vi "2017RefLoopPulseGen_Summer.vi"() -> ()   [LabVIEW 2015]
uses:
  Utility Sub VIs/pulse_generator_controls_multiheater_refnums.ctl
  Stop_Global_Variable.vi
  Utility Sub VIs/pulse_generator_data_controls_refnums.ctl
  Utility Sub VIs/pulse_generator_data_refnums.ctl
  Utility Sub VIs/pulse_generator_data_charts_refnums.ctl
  <vilib>/addons/control/pid/NI_PID_autopid.lvlib
  <vilib>/Utility/error.llb/DialogType.ctl
  <vilib>/DAQmx/configure/task.llb/DAQmx Configure Watchdog Expiration States (Counter Output).vi
  <vilib>/DAQmx/read.llb/DAQmx Read (Analog 1D Wfm NChan NSamp).vi
  <vilib>/DAQmx/configure/task.llb/DAQmx Configure Watchdog Expiration States (Analog Output).vi
  Utility Sub VIs/pulse_generator_data.ctl
  Utility Sub VIs/pulse_generator_data_controls.ctl
  Utility Sub VIs/pulse_generator_data_charts.ctl
  Utility Sub VIs/pulse_generator_multiheater_controls.ctl
  Input Channel Lists/test_section_physical_channels.ctl
  Input Channel Lists/pg_control_physical_channels.ctl
  Input Channel Lists/watchdog_config_channels.ctl
  Input Channel Lists/valve_physical_channels.ctl
  Utility Sub VIs/valve_pid_control.ctl
  Input Channel Lists/float_switch_physical_channels.ctl
  Input Channel Lists/pulse_generator_input_physical_channels.ctl
panel:
  out "dP Queue":refnum<queue>
  out "loopDataQueue":refnum<queue>
  out "Float 4":bool
  out "Float 3":bool
  out "Float 2":bool
  out "Float 1":bool
  out "Pulse Generator":u8(slide) scale=0.0..100.0 scale format="%.0f%"
  out "autoOffsetPsatQueue":refnum<queue>
  out "start time":timestamp
  out "Seconds Since\nSession Start":dbl
  out "dP Recording Progress":u32(slide) scale=0.0..10000.0
  out "dP Data Index":dbl
  out "Loop Data Index":dbl
  in  "dP Data Prefix":string
  in  "dP Data Folder":path
  in  "Loop Data Prefix":string
  in  "Loop Data Folder":path
  in  "Record dP Data":bool
  in  "Record Loop Data":bool
  out "dP Data Labels":string[](array[string])=["Vap Mass Flow", "Liq Mass Flow", "DP", "Liq Tank P", "LiqTank T", "Sep P", "SepT", "Liq In P", "Liq In T", "Vap Tank P", "Vap Tank T", "Dev Section P", "Dev Section T", "Up TS P", "Up TS T", "Low TS P", "Low TS T", "Cond Top T", "Evap Top T", "Cond Bot T", "Evap Bot T", "Win 3-4 P", "Top Heat T", "Bot Heat T"]
  out "Time Stamp":timestamp format="%<%H:%M:%S%1u>T"
  out "Loop Data Labels":string[](array[string])=["Vap Mass Flow", "Liq Mass Flow", "DP", "Liq Tank P", "LiqTank T", "Sep P", "SepT", "Liq In P", "Liq In T", "Vap Tank P", "Vap Tank T", "Dev Section P", "Dev Section T", "Up TS P", "Up TS T", "Low TS P", "Low TS T", "Cond Top T", "Evap Top T", "Cond Bot T", "Evap Bot T", "Win 3-4 P", "Top Heat T", "Bot Heat T"]
  in  "Tab Control":T1(tab)
  out "Auto Offset Progress":u32(slide) scale=0.0..20.0
  out "Pressure/Temperature/Mixture Properties":T2
  in  "Offset Parameters":T3={"Separator \nTemperature"=0.0, "Separator Pressure"=0.0, "Lower Test Section\nTemperature"=0.0, "Lower Test Section\nPressure"=0.0, "Vapor Tank (Top) \nHeater"=0.0, "Liquid Tank (Bottom) \nHeater"=0.0, "Vapor Tank\nTemperature Offset"=0.0, "Vapor Tank\nPressure "=0.0, "Upper Test Section\nTemperature"=0.0, "Upper Test Section\nPressure"=0.0, "Vapor Inlet \nTemperature"=0.0, "Dev Section\nPressure"=0.0, "Liquid Tank\nTemperature"=0.0, "Liquid Tank\nPressure"=0.0, "Liquid Inlet\nTemperature "=0.0, "Liquid Inlet\nPressure"=0.0, "Atmospheric Pressure [Pa]"=101325.0}
  in  "Auto Offset":bool
  out "# of Averages Processed":i32
  out "Dynamic Data Type":dynamicdata(graph)
  out "Vapor Mass Flow Rate":dynamicdata(graph)
  out "Liquid Mass Flow Rate":dynamicdata(graph)
  out "Vapor Flow Data":T4
  out "Liquid Flow Data":T5
  in  "Liquid PID Control":T6={"proportional gain (Kc)"=1.0, "integral time (Ti, min)"=0.01, "derivative time (Td, min)"=0.0, "Valve Voltage [V]"=0.0, "Min % Open"=2.0, "Max % Open"=3.0, "Reinitialize?"=FALSE, "Valve On/Off"=FALSE, "Mode"=FALSE, "Full Flow Rate"=0.0, "Flow Set Point [g/s]"=0.0, "AutoTune"=FALSE} {"Flow Set Point [g/s]" format="%.2f"; "Full Flow Rate" format="%.2f"; "Max % Open" min=0.0 max=100.0 format="%.2f"; "Min % Open" min=0.0 max=100.0 format="%.2f"; "Valve Voltage [V]" format="%.2f"; "derivative time (Td, min)" format="%.3f"; "integral time (Ti, min)" format="%.3f"; "proportional gain (Kc)" format="%.3f"}
  in  "Vapor PID Control":T6={"proportional gain (Kc)"=1.0, "integral time (Ti, min)"=0.01, "derivative time (Td, min)"=0.0, "Valve Voltage [V]"=0.0, "Min % Open"=2.0, "Max % Open"=3.0, "Reinitialize?"=FALSE, "Valve On/Off"=FALSE, "Mode"=FALSE, "Full Flow Rate"=0.0, "Flow Set Point [g/s]"=0.0, "AutoTune"=FALSE} {"Flow Set Point [g/s]" format="%.2f"; "Full Flow Rate" format="%.2f"; "Max % Open" min=0.0 max=100.0 format="%.2f"; "Min % Open" min=0.0 max=100.0 format="%.2f"; "Valve Voltage [V]" format="%.2f"; "derivative time (Td, min)" format="%.3f"; "integral time (Ti, min)" format="%.3f"; "proportional gain (Kc)" format="%.3f"}
  in  "Pulse Generator Offsets & Data Saving Controls":T7={"PG-TS Offset"=11500.0, "Pitot Offset"=0.0, "PG Abs Offset"=11500.0, "Sampling\nFrequency"=1000.0, "Recording Duration"=10.0}
  out "Pulse Generator Measurements":T8={"PG to TS dP"=4351.8068090218785, "PG Abs"=119484.80284900061, "Mass Flow Rate"=nan, "Pitot dP"=-4308.9404273994505, "Pitot Amps"=2.6415199999999147e-07, "Vapor Temperature"=19.805676371442082, "Liquid Temperature"=19.52526901660894, "Vapor Sat Pressure"=121.24568157832624, "Liquid Sat Pressure"=119.96937909943745, "W1-4 dP[Pa]"=19.52526901660894, "W1-7 dP[Pa]"=119.96937909943745}
  out "Pulse Generator Charts":T9={" Camera Voltage"=9.650720988784618, "Pitot dP"=-0.0006103608758678569, "Absolute Tank Pressure"=119484.80284900061, "Pulse Generator to Test Section dP"=11360.460004869077}
  in  "Commit Settings":bool
  in  "Settings Subpanel":enum32{"Input", "Output", "Safety"}(tab)
  in  "Input":T13={"Test Section Physical Channels"={"Vapor Mass Flow Current"="cDAQ1Mod1/ai10", "Vapor Line Density Current"="cDAQ1Mod1/ai11", "Liquid Mass Flow Current"="cDAQ1Mod1/ai8", "Liquid Line Density Current"="cDAQ1Mod1/ai9", "Vapor Tank Pressure"="cDAQ1Mod1/ai3", "Liquid Tank Pressure"="cDAQ1Mod1/ai2", "Separator Pressure"="cDAQ1Mod1/ai4", "Liquid Inlet Pressure"="cDAQ1Mod1/ai0", "Dev Section Pressure"="cDAQ1Mod1/ai1", "Vapor Tank Temperature"="cDAQ1Mod6/ai2", "Vapor Inlet Temperature"="cDAQ1Mod6/ai0", "Liquid Tank Temperature"="cDAQ1Mod6/ai3", "Liquid Inlet Temperature"="cDAQ1Mod6/ai4", "Separator Temperature"="cDAQ1Mod6/ai1", "Lower Test Section Pressure"="cDAQ1Mod1/ai5", "Lower Test Section Temperature"="cDAQ1Mod6/ai5", "Top Heater Temperature"="cDAQ1Mod6/ai6", "Bottom Heater Temperature"="cDAQ1Mod6/ai7", "Pressure Drop"="cDAQ1Mod1/ai12", "Upper Test Section Temperature"="cDAQ1Mod6/ai9", "Upper Test Section Pressure"="cDAQ1Mod1/ai7", "Condenser Top Temperature"="cDAQ1Mod6/ai8", "Condenser Bottom Temperature"="cDAQ1Mod6/ai10", "Evaporator Top Temperature"="cDAQ1Mod6/ai11", "Evaporator Bottom Temperature"="cDAQ1Mod6/ai12", "Test Section Window 3-4 Pressure"="cDAQ1Mod1/ai6"}, "Float Switch Physical Channels"={"Float Line 1"="", "Float Line 2"="", "Float Line 3"="", "Float Line 4"=""}, "Pulse Generator Input Physical Channels"={"Absolute Pressure"="cDAQ1Mod5/ai1", "PG to TS dP"="cDAQ1Mod5/ai0", "Pitot dP"="cDAQ1Mod3/ai6", "PG Temperature 1"="cDAQ1Mod7/ai0", "PG Temperature 2"="cDAQ1Mod7/ai1", "dP Windows 1 to 7"="cDAQ1Mod1/ai2", "dP Windows 1 to 4"="cDAQ1Mod3/ai3", "Camera Votlage"="cDAQ1Mod2/ai0"}}
  in  "Output":T16={"Pulse Generator Control Physical Channels"={"1000W 1"="Dev1/port1/line0", "1000W 2"="Dev1/port1/line1", "1000W 3"="Dev1/port1/line2", "500W 1"="Dev1/port1/line3", "250W 1"="cDAQ1Mod8/ctr0", "125W 1 Var"="cDAQ1Mod8/ctr0", "125W Variable/Fixed"="Fixed", "125W 1 Fix"="cDAQ1Mod8/ctr0", "Counter Line"="cDAQ1Mod8/ctr0", "Direction Line"="cDAQ1Mod8/ctr0"}, "Vapor/Liquid Valve Physical Channels"={"Vapor Valve"="cDAQ1Mod4/ao2", "Liquid Valve"="cDAQ1Mod4/ao3"}}
  in  "Safety":T17
  in  "Watchdog Configurations":T18 {"Counter Outputs"."expiration state" items=["Low"=10214, "High"=10192, "No Change"=10160]; "Analog Outputs"."output type" items=["Voltage"=10322, "Current"=10134, "No Change"=10160]; "Digital Outputs"."expiration state" items=["High"=10192, "Low"=10214, "Tristate"=10310, "No Change"=10160]}
  out "System Running":bool
  in  "Pulse Train, Steam Heater Controls":T19={"Start Pulse"=FALSE, "Stop Pulse"=FALSE, "Pulse Gen\nActive?"=FALSE, "Frequency (Hz)"=3000.0, "Duty Cycle"=0.5, "Idle State"=10214, "Steps"=1000, "Stepper Motor Direction"=FALSE, "Heaters"=FALSE, "Heater ON?"=FALSE, "1000-1"=FALSE, "1000-2"=FALSE, "1000-3"=FALSE, "500-1"=FALSE, "250-1"=FALSE, "125W Duty Cycle"=0.5, "125W Frequency (Hz)"=1000.0, "125-1"=FALSE} {"125W Frequency (Hz)" min=0.0; "125W Duty Cycle" min=0.0; "Frequency (Hz)" min=1.0 step=500.0; "Duty Cycle" min=0.1 max=0.99 step=0.1; "Idle State" items=["High"=10192, "Low"=10214]}
  out "error out":errorcluster
  out "Loop Time [ms]":u32
  in  "Stop":bool
  # "Saturation\nPressure [Pa]"
  # "Saturation\nTemperature [C]"
  # "Pressure [Pa]"
  # "Temperature [C]"
  # "Streamwise(dP)"
  # "Liquid Tank"
  # "Separator"
  # "Liquid Inlet"
  # "Vapor Tank"
  # "Vapor Inlet\n(Dev Section)"
  # "Upper Test Section"
  # "Lower Test Section"
  # "Offsets"
  # "Pulse Generator - Test Section dP"
  # "Pulse Generator Absolute Pressure"
  # "Pitot dP"
  # "Pitot Current"
  # "Mass Flow Rate"
  # "Heater Lines and Switches"
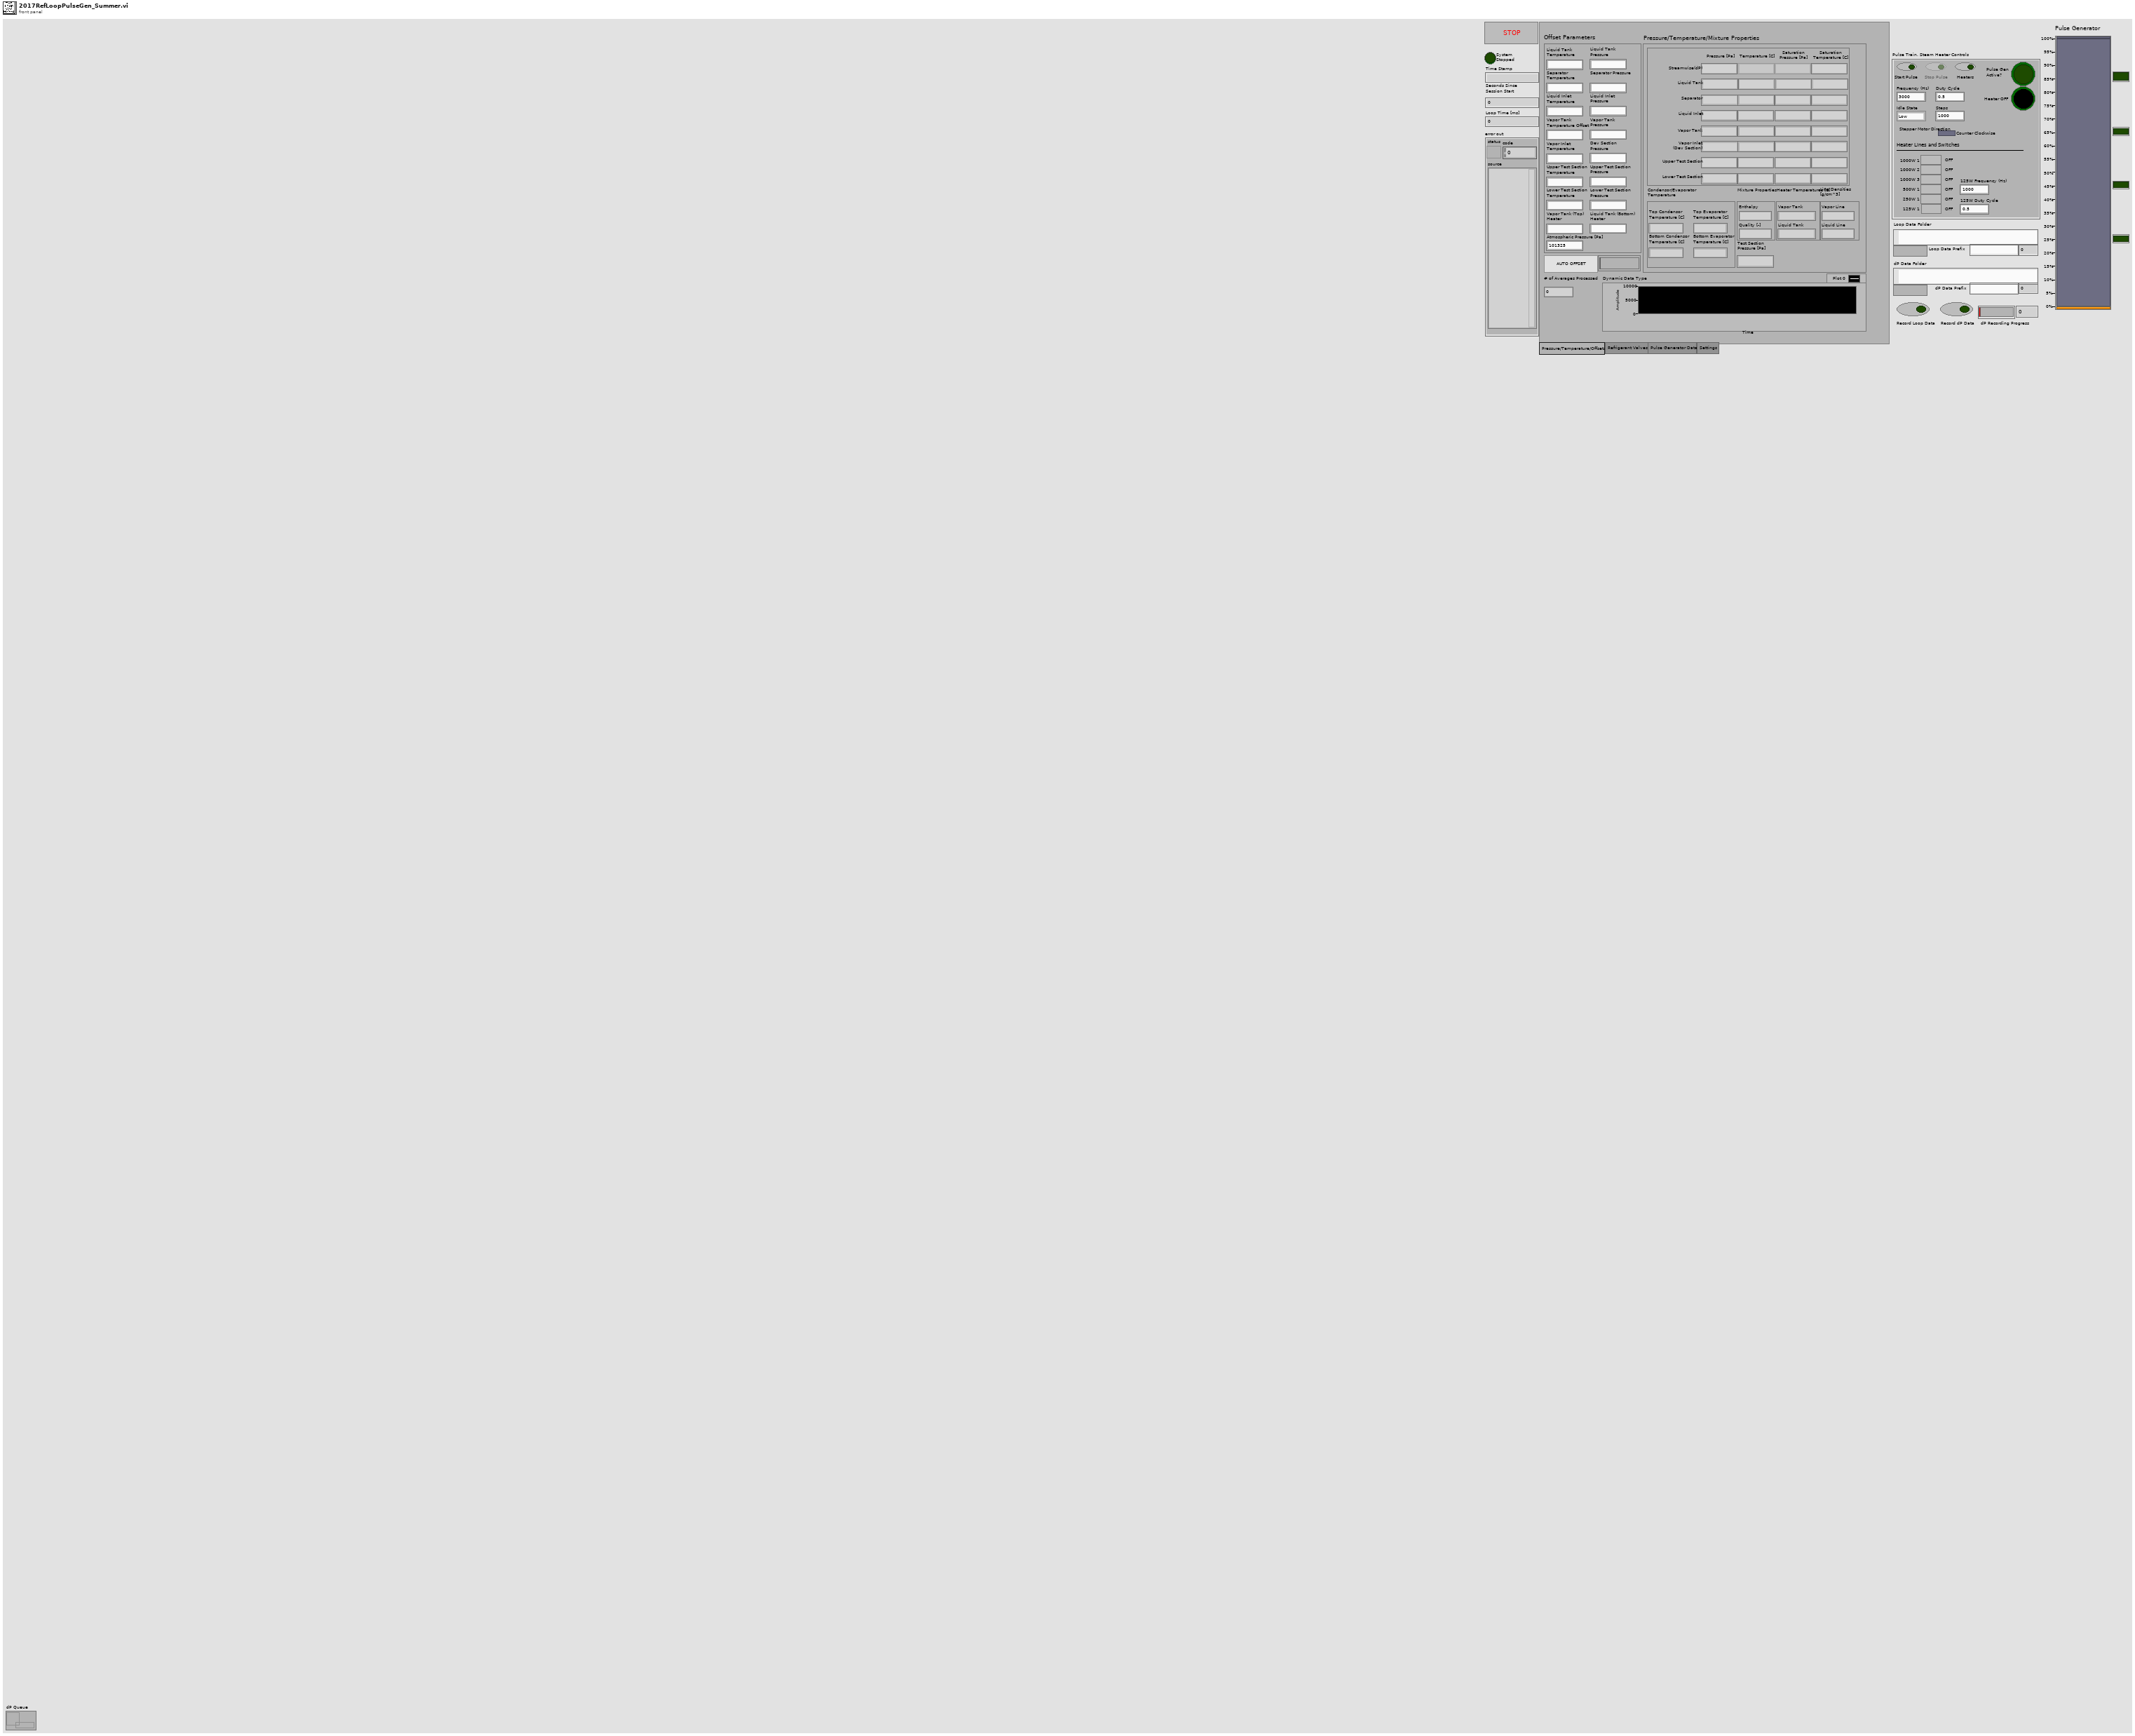
[diagram p1: front panel]
types:
  T1 = enum32{"Pressure/Temperature/Offsets", "Refrigerant Valves", "Pulse Generator Data", "Settings"}
  T2 = cluster{"Line Densities\n[g/cm^3]":cluster{"Vapor Line":dbl, "Liquid Line":dbl}, "Mixture Properties":cluster{"Enthalpy":dbl, "Quality [-]":dbl}, "[Readings]":cluster{"Streamwise P":dbl, "Streamwise T":dbl, "Streamwise Sat P":dbl, "Streamwise Sat T":dbl, "Liquid Tank P":dbl, "Liquid Tank T":dbl, "Liquid Tank Sat P":dbl, "Liquid Tank Sat T":dbl, "Separator P":dbl, "Separator T":dbl, "Separator Sat P":dbl, "Separator Sat T":dbl, "Liquid Inlet P":dbl, "Liquid Inlet T":dbl, "Liquid Inlet Sat P":dbl, "Liquid Inlet Sat T":dbl, "Vapor Tank P":dbl, "Vapor Tank T":dbl, "Vapor Tank Sat P":dbl, "Vapor Tank Sat T":dbl, "Vapor Inlet P":dbl, "Vapor Inlet T":dbl, "Vapor Inlet Sat P":dbl, "Vapor Inlet Sat T":dbl, "Upper Test Section P":dbl, "Upper Test Section T":dbl, "Upper Test Section Sat P":dbl, "Upper Test Section Sat T":dbl, "Lower Test Section P":dbl, "Lower Test Section T":dbl, "Lower Test Section Sat P":dbl, "Lower Test Section Sat T":dbl}, "Condensor/Evaporator\nTemperature":cluster{"Bottom Evaporator\nTemperature [C]":dbl, "Bottom Condensor\nTemperature [C]":dbl, "Top Evaporator\nTemperature [C]":dbl, "Top Condensor\nTemperature [C]":dbl}, "Test Section \nPressure [Pa]":dbl, "Heater Temperatures [C]":cluster{"Vapor Tank":dbl, "Liquid Tank":dbl}}
  T3 = cluster{"Separator \nTemperature":dbl, "Separator Pressure":dbl, "Lower Test Section\nTemperature":dbl, "Lower Test Section\nPressure":dbl, "Vapor Tank (Top) \nHeater":dbl, "Liquid Tank (Bottom) \nHeater":dbl, "Vapor Tank\nTemperature Offset":dbl, "Vapor Tank\nPressure ":dbl, "Upper Test Section\nTemperature":dbl, "Upper Test Section\nPressure":dbl, "Vapor Inlet \nTemperature":dbl, "Dev Section\nPressure":dbl, "Liquid Tank\nTemperature":dbl, "Liquid Tank\nPressure":dbl, "Liquid Inlet\nTemperature ":dbl, "Liquid Inlet\nPressure":dbl, "Atmospheric Pressure [Pa]":dbl}
  T4 = cluster{"Vapor Flow rate [g/s]":dbl, "Line Density [g/cm^3]":dbl}
  T5 = cluster{"Liquid Flow rate [g/s]":dbl, "Line Density [g/cm^3]":dbl}
  T6 = typedef "valve_pid_control.ctl" = cluster{"proportional gain (Kc)":dbl, "integral time (Ti, min)":dbl, "derivative time (Td, min)":dbl, "Valve Voltage [V]":dbl, "Min % Open":dbl, "Max % Open":dbl, "Reinitialize?":bool, "Valve On/Off":bool, "Mode":bool, "Full Flow Rate":dbl, "Flow Set Point [g/s]":dbl, "AutoTune":bool}
  T7 = typedef "pulse_generator_data_controls.ctl" = cluster{"PG-TS Offset":dbl, "Pitot Offset":dbl, "PG Abs Offset":dbl, "Sampling\nFrequency":dbl, "Recording Duration":dbl}
  T8 = typedef "pulse_generator_data.ctl" = cluster{"PG to TS dP":dbl, "PG Abs":dbl, "Mass Flow Rate":dbl, "Pitot dP":dbl, "Pitot Amps":dbl, "Vapor Temperature":dbl, "Liquid Temperature":dbl, "Vapor Sat Pressure":dbl, "Liquid Sat Pressure":dbl, "W1-4 dP[Pa]":dbl, "W1-7 dP[Pa]":dbl}
  T9 = typedef "pulse_generator_data_charts.ctl" = cluster{" Camera Voltage":dbl, "Pitot dP":dbl, "Absolute Tank Pressure":dbl, "Pulse Generator to Test Section dP":dbl}
  T10 = typedef "test_section_physical_channels.ctl" = cluster{"Vapor Mass Flow Current":tag, "Vapor Line Density Current":tag, "Liquid Mass Flow Current":tag, "Liquid Line Density Current":tag, "Vapor Tank Pressure":tag, "Liquid Tank Pressure":tag, "Separator Pressure":tag, "Liquid Inlet Pressure":tag, "Dev Section Pressure":tag, "Vapor Tank Temperature":tag, "Vapor Inlet Temperature":tag, "Liquid Tank Temperature":tag, "Liquid Inlet Temperature":tag, "Separator Temperature":tag, "Lower Test Section Pressure":tag, "Lower Test Section Temperature":tag, "Top Heater Temperature":tag, "Bottom Heater Temperature":tag, "Pressure Drop":tag, "Upper Test Section Temperature":tag, "Upper Test Section Pressure":tag, "Condenser Top Temperature":tag, "Condenser Bottom Temperature":tag, "Evaporator Top Temperature":tag, "Evaporator Bottom Temperature":tag, "Test Section Window 3-4 Pressure":tag}
  T11 = typedef "float_switch_physical_channels.ctl" = cluster{"Float Line 1":tag, "Float Line 2":tag, "Float Line 3":tag, "Float Line 4":tag}
  T12 = typedef "pulse_generator_input_physical_channels.ctl" = cluster{"Absolute Pressure":tag, "PG to TS dP":tag, "Pitot dP":tag, "PG Temperature 1":tag, "PG Temperature 2":tag, "dP Windows 1 to 7":tag, "dP Windows 1 to 4":tag, "Camera Votlage":tag}
  T13 = cluster{"Test Section Physical Channels":T10, "Float Switch Physical Channels":T11, "Pulse Generator Input Physical Channels":T12}
  T14 = typedef "pg_control_physical_channels.ctl" = cluster{"1000W 1":tag, "1000W 2":tag, "1000W 3":tag, "500W 1":tag, "250W 1":tag, "125W 1 Var":tag, "125W Variable/Fixed":string, "125W 1 Fix":tag, "Counter Line":tag, "Direction Line":tag}
  T15 = typedef "valve_physical_channels.ctl" = cluster{"Vapor Valve":tag, "Liquid Valve":tag}
  T16 = cluster{"Pulse Generator Control Physical Channels":T14, "Vapor/Liquid Valve Physical Channels":T15}
  T17 = cluster{"Pulse Generator Safety Values":cluster{"Absolute Pulse Generator Pressure Limit":dbl, "Seconds Allowed Pulse Generator Excess Pressure":dbl, "Absolute Pulse Generator Temperature Limit":dbl}}
  T18 = typedef "watchdog_config_channels.ctl" = cluster{"Task Name":string, "DAQmx Device Name":tag, "Digital Outputs":cluster{"physical channel":tag, "expiration state":u16}[], "Analog Outputs":cluster{"physical channel":tag, "value":dbl, "output type":i32}[], "Counter Outputs":cluster{"physical channel":tag, "expiration state":u16}[]}[]
  T19 = typedef "pulse_generator_multiheater_controls.ctl" = cluster{"Start Pulse":bool, "Stop Pulse":bool, "Pulse Gen\nActive?":bool, "Frequency (Hz)":dbl, "Duty Cycle":dbl, "Idle State":i32, "Steps":i32, "Stepper Motor Direction":bool, "Heaters":bool, "Heater ON?":bool, "1000-1":bool, "1000-2":bool, "1000-3":bool, "500-1":bool, "250-1":bool, "125W Duty Cycle":dbl, "125W Frequency (Hz)":dbl, "125-1":bool}
  T20 = cluster{"Vapor Flow rate [g/s]":dbl, "Liquid Flow rate [g/s]":dbl, "Pressure/Temperature/Mixture Properties":cluster{"Line Densities\n[g/cm^3]":cluster{"Vapor Line":dbl, "Liquid Line":dbl}, "Mixture Properties":cluster{"Enthalpy":dbl, "Quality [-]":dbl}, "[Readings]":cluster{"Streamwise P":dbl, "Streamwise T":dbl, "Streamwise Sat P":dbl, "Streamwise Sat T":dbl, "Liquid Tank P":dbl, "Liquid Tank T":dbl, "Liquid Tank Sat P":dbl, "Liquid Tank Sat T":dbl, "Separator P":dbl, "Separator T":dbl, "Separator Sat P":dbl, "Separator Sat T":dbl, "Liquid Inlet P":dbl, "Liquid Inlet T":dbl, "Liquid Inlet Sat P":dbl, "Liquid Inlet Sat T":dbl, "Vapor Tank P":dbl, "Vapor Tank T":dbl, "Vapor Tank Sat P":dbl, "Vapor Tank Sat T":dbl, "Vapor Inlet P":dbl, "Vapor Inlet T":dbl, "Vapor Inlet Sat P":dbl, "Vapor Inlet Sat T":dbl, "Upper Test Section P":dbl, "Upper Test Section T":dbl, "Upper Test Section Sat P":dbl, "Upper Test Section Sat T":dbl, "Lower Test Section P":dbl, "Lower Test Section T":dbl, "Lower Test Section Sat P":dbl, "Lower Test Section Sat T":dbl}, "Condensor/Evaporator\nTemperature":cluster{"Bottom Evaporator\nTemperature [C]":dbl, "Bottom Condensor\nTemperature [C]":dbl, "Top Evaporator\nTemperature [C]":dbl, "Top Condensor\nTemperature [C]":dbl}, "Test Section \nPressure [Pa]":dbl, "Heater Temperatures [C]":cluster{"Vapor Tank":dbl, "Liquid Tank":dbl}}, "Seconds Since \nSession Start":dbl}
  T21 = enum8{"Enabled", "Disabled", "Disabled and Grayed Out"}
  T22 = typedef "DialogType.ctl" = u16
  T23 = cluster{"physical channel":tag, "expiration state":u16}[]
  T24 = cluster{"physical channel":tag, "value":dbl, "output type":i32}[]
  T25 = cluster{"Vapor Flow rate [g/s]":dbl, "Liquid Flow rate [g/s]":dbl, "Pressure/Temperature/Mixture Properties":cluster{"Line Densities\n[g/cm^3]":cluster{"Vapor Line":dbl, "Liquid Line":dbl}, "Mixture Properties":cluster{"Enthalpy":dbl, "Quality [-]":dbl}, "[Readings]":cluster{"Streamwise P":dbl, "Streamwise T":dbl, "Streamwise Sat P":dbl, "Streamwise Sat T":dbl, "Liquid Tank P":dbl, "Liquid Tank T":dbl, "Liquid Tank Sat P":dbl, "Liquid Tank Sat T":dbl, "Separator P":dbl, "Separator T":dbl, "Separator Sat P":dbl, "Separator Sat T":dbl, "Liquid Inlet P":dbl, "Liquid Inlet T":dbl, "Liquid Inlet Sat P":dbl, "Liquid Inlet Sat T":dbl, "Vapor Tank P":dbl, "Vapor Tank T":dbl, "Vapor Tank Sat P":dbl, "Vapor Tank Sat T":dbl, "Vapor Inlet P":dbl, "Vapor Inlet T":dbl, "Vapor Inlet Sat P":dbl, "Vapor Inlet Sat T":dbl, "Upper Test Section P":dbl, "Upper Test Section T":dbl, "Upper Test Section Sat P":dbl, "Upper Test Section Sat T":dbl, "Lower Test Section P":dbl, "Lower Test Section T":dbl, "Lower Test Section Sat P":dbl, "Lower Test Section Sat T":dbl}, "Condensor/Evaporator\nTemperature":cluster{"Bottom Evaporator\nTemperature [C]":dbl, "Bottom Condensor\nTemperature [C]":dbl, "Top Evaporator\nTemperature [C]":dbl, "Top Condensor\nTemperature [C]":dbl}, "Test Section \nPressure [Pa]":dbl, "Heater Temperatures [C]":cluster{"Vapor Tank":dbl, "Liquid Tank":dbl}}, "Seconds Since\nSession Start":dbl}
  T26 = cluster{"proportional gain (Kc)":dbl, "integral time (Ti, min)":dbl, "derivative time (Td, min)":dbl}
  T27 = typedef "pulse_generator_data_charts_refnums.ctl" = cluster{"Pulse Generator to Test Section dP":refnum<vi>, "Pitot dP":refnum<vi>, "Abs Tank Pressure":refnum<vi>, "Camera Voltage":refnum<vi>}
  T28 = typedef "pulse_generator_data_refnums.ctl" = cluster{"Vapor Temperature":refnum<vi>, "Vapor Sat Pressure":refnum<vi>, "Liquid Temperature":refnum<vi>, "Liquid Sat Pressure":refnum<vi>, "PG to TS dP":refnum<vi>, "Pitot Current":refnum<vi>, "Pitot dP":refnum<vi>, "Mass Flow Rate":refnum<vi>, "PG Abs Pressure":refnum<vi>, "W1-4 dP":refnum<vi>, "W1-7 dP":refnum<vi>}
  T29 = typedef "pulse_generator_data_controls_refnums.ctl" = cluster{"PG Abs Offset":refnum<vi>, "Pitot Offset":refnum<vi>, "PG-TS Offset":refnum<vi>, "Recording Duration":refnum<vi>, "Sampling Rate":refnum<vi>}
  T30 = typedef "pulse_generator_controls_multiheater_refnums.ctl" = cluster{"Start Pulse":refnum<vi>, "Stop Pulse":refnum<vi>, "Heaters":refnum<vi>, "Counter":refnum<vi>, "Frequency (Hz)":refnum<vi>, "Duty Cycle":refnum<vi>, "Idle State":refnum<vi>, "Pulse Generator Active":refnum<vi>, "Stepper Motor Direction":refnum<vi>, "Steps":refnum<vi>, "Direction Line":refnum<vi>, "1000-1 Line":refnum<vi>, "1000-2 Line":refnum<vi>, "1000-3 Line":refnum<vi>, "500-1 Line":refnum<vi>, "250-1 Line":refnum<vi>, "125-1 Line Var":refnum<vi>, "1000-1":refnum<vi>, "1000-2":refnum<vi>, "1000-3":refnum<vi>, "500-1":refnum<vi>, "250-1":refnum<vi>, "125-1":refnum<vi>, "125W Frequency (Hz)":refnum<vi>, "125W Duty Cycle":refnum<vi>, "Heater ON?":refnum<vi>, "125-1 Line Fix":refnum<vi>}
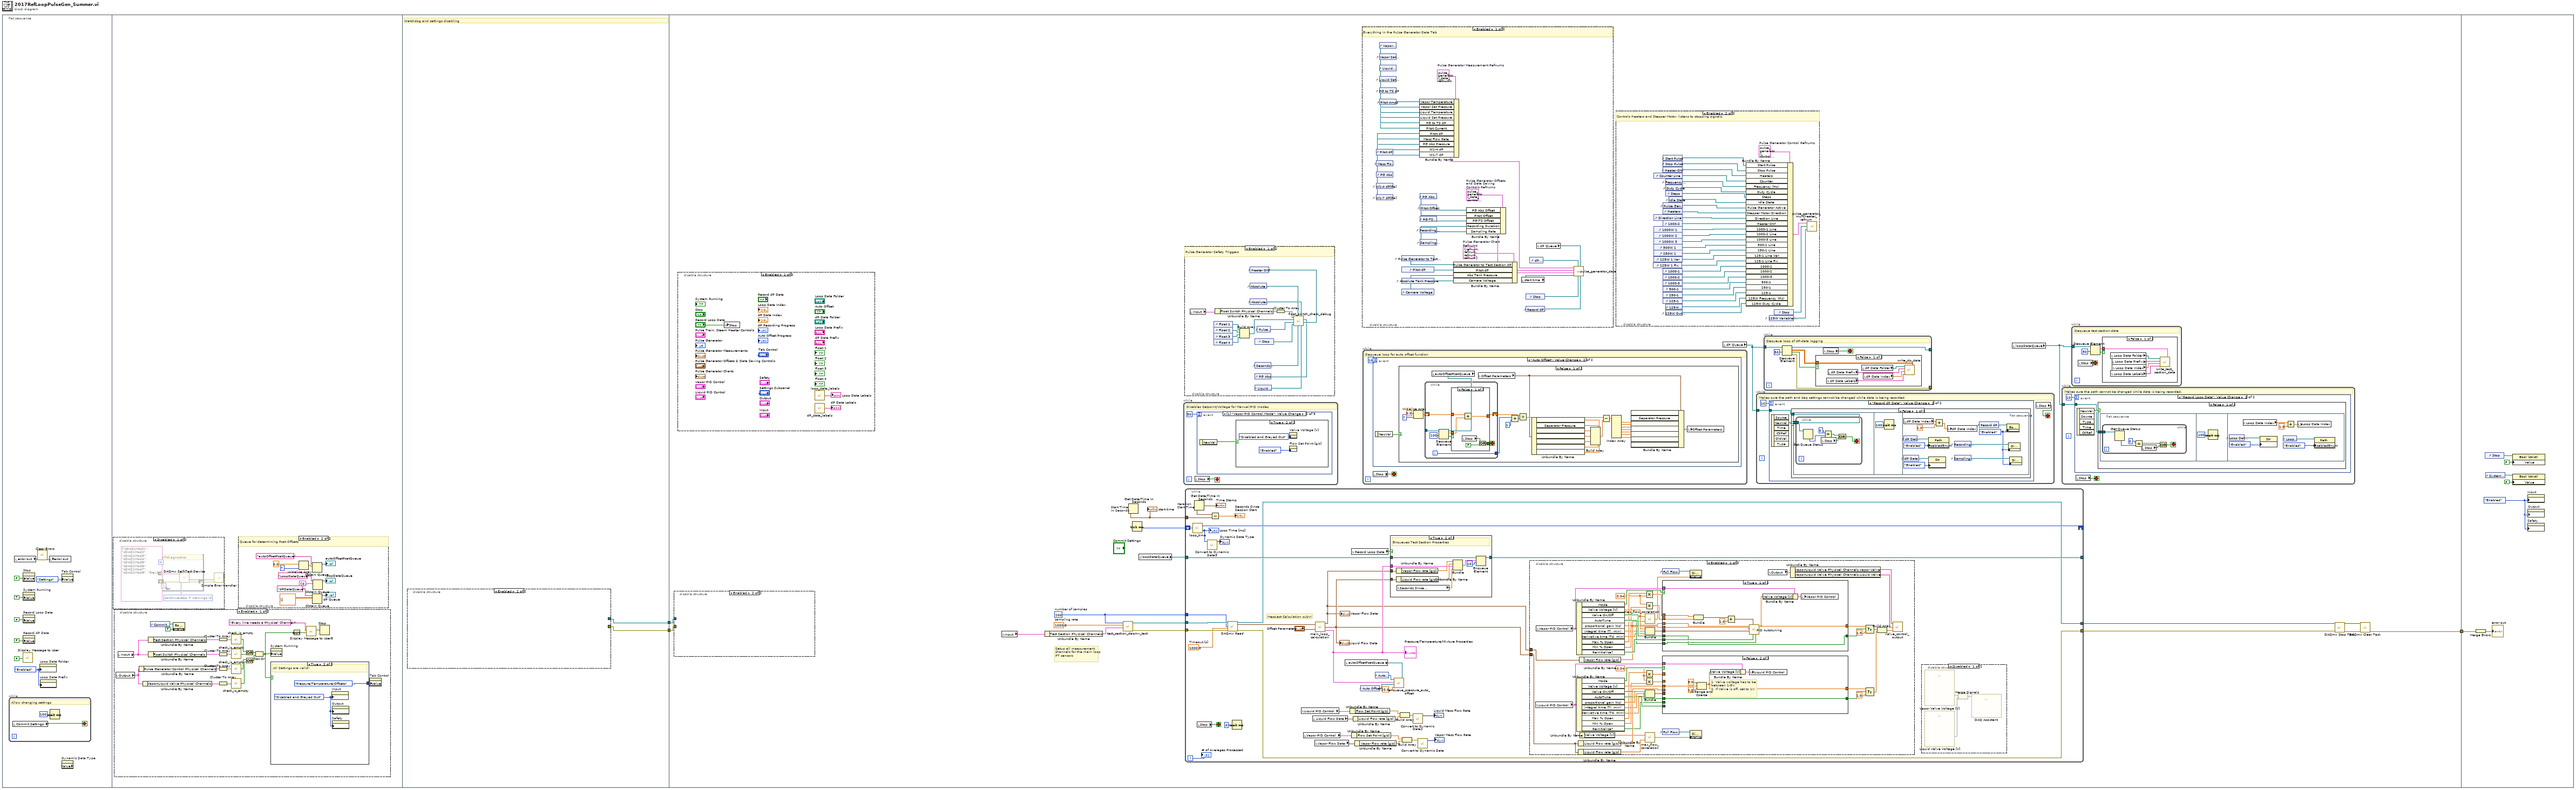
[diagram p0: block diagram]
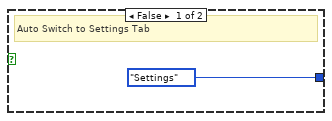
[diagram p3: hidden frame]
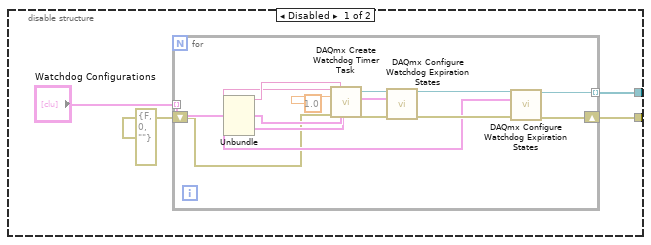
[diagram p6: hidden frame]
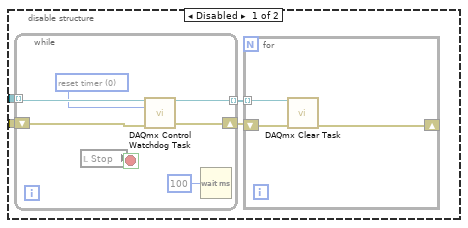
[diagram p11: hidden frame]
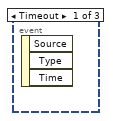
[diagram p12: hidden frame]
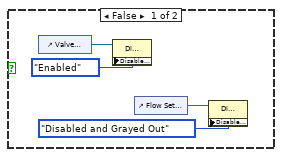
[diagram p13: hidden frame]
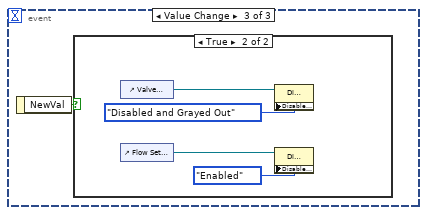
[diagram p14: hidden frame]
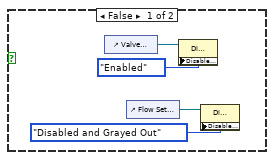
[diagram p15: hidden frame]
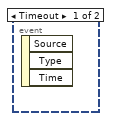
[diagram p16: hidden frame]
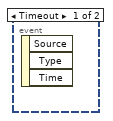
[diagram p19: hidden frame]
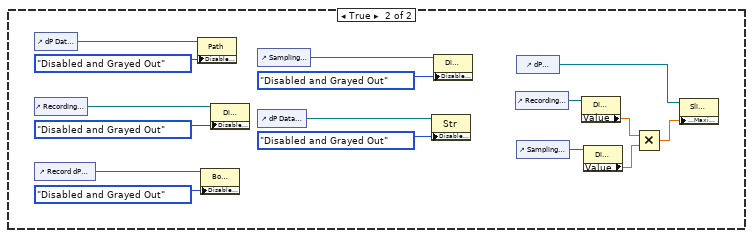
[diagram p20: hidden frame]
diagram:
  n1 = flat-sequence {
    tunnel: [w59] -> w2
    tunnel: [w58] -> w1
    tunnel: [w91] -> w3
    tunnel: w2 -> [w85]
    tunnel: w1 -> [w84]
    tunnel: w3 -> [w492]
    frame #0 {
      w4 = T21."Enabled" ("Disabled")
      n2 = while {
        stop <- w13 stop-if-true
        # "Allow changing settings"
        n3 = local read "Commit Settings"() -> (w13:bool)
        n4 = Wait (ms)(milliseconds to wait=u32 100) -> ()  [unwired: 1 out]
      }
      n5 = local read "error out"() -> (w12:errorcluster)
      n6 = call "Display Message to User"("Enable"=FALSE) -> ()  [unwired: 9 in, 2 out]
      n7 = property on="Stop" class="Bool (strict)"("Value"=FALSE) -> ()  [unwired: 2 in, 2 out]
      n8 = property on="System Running" class="Bool (strict)"("Value"=TRUE) -> ()  [unwired: 2 in, 2 out]
      n9 = property on="Record Loop Data" class="Bool (strict)"("Value"=FALSE) -> ()  [unwired: 2 in, 2 out]
      n10 = property on="Record dP Data" class="Bool (strict)"("Value"=FALSE) -> ()  [unwired: 2 in, 2 out]
      n11 = call <vilib>:"Clear Errors.vi"("error in (no error)"=w12) -> ("error out"=w10:errorcluster)  [unwired: 5 in, 1 out]
      n12 = property on="Loop Data Folder" class="Path"("DisabledEnum"=w4) -> ()  [unwired: 2 in, 2 out]
      n13 = property on="Loop Data Prefix" class="Str"("DisabledEnum"=w4) -> ()  [unwired: 2 in, 2 out]
      n14 = local write "error out"(w10) -> ()
      n15 = property on="Tab Control" class="TabCtl (strict)"("Value"=T1."Settings" ("Tab Control")) -> ()  [unwired: 2 in, 2 out]
      n16 = property on="Dynamic Data Type" class="WFChart (strict)" props=["Value"]() -> ()  [unwired: 2 in, 3 out]
    }
    frame #1 {
      n17 = disable-structure shown="Disabled" {
        frame Disabled {
          w52 = T22 4 items=["no dialog", "OK message", "continue or stop message", "OK message + warnings", "continue/stop + warnings"] ("type of dialog (OK msg:1)")
          n18 = for {
            tunnel: string[] ["cDAQ1Mod1", "cDAQ1Mod2", "cDAQ1Mod3", "cDAQ1Mod4", "cDAQ1Mod5", "cDAQ1Mod6", "cDAQ1Mod7", "cDAQ1Mod8", "Dev1"] -> [w57] mode=indexing
            shift-right: [w56] -> w53
            shift-left: _ -> [w55]
            # "Self-Diagnostics"
            n19 = call <vilib>:"DAQmx Self-Test Device.vi"("device in"=w57, "error in"=w55) -> ("error out"=w56:errorcluster)  [unwired: 13 in]
          }
          n20 = call <vilib>:"Simple Error Handler.vi"("type of dialog (OK msg:1)"=w52, "error in (no error)"=w53) -> ()  [unwired: 3 in, 5 out]
        }
        frame Enabled {
        }
      }
      n21 = disable-structure shown="Enabled" {
        frame Enabled {
          n22 = local read "Output"() -> (w26:T16)
          n23 = local read "Input"() -> (w32:T13)
          n24 = Unbundle By Name(w26) -> ("Pulse Generator Control Physical Channels"=w33:T14)
          n25 = Unbundle By Name(w26) -> ("Vapor/Liquid Valve Physical Channels"=w31:T15)
          n26 = Unbundle By Name(w32) -> ("Test Section Physical Channels"=w35:T10)
          n27 = Unbundle By Name(w32) -> ("Float Switch Physical Channels"=w34:T11)
          n28 = control-ref of="Commit Settings"() -> (w29:refnum<vi>)
          n29 = property class="Bool (strict)"(reference=w29, "Value"=FALSE ("Commit Settings")) -> ()  [unwired: 1 in, 2 out]
          n30 = Cluster To Array(cluster=w35) -> (array=w48:tag[])
          n31 = Cluster To Array(cluster=w34) -> (array=w47:tag[])
          n32 = Cluster To Array(cluster=w33) -> (array=w44:string[])
          n33 = Cluster To Array(cluster=w31) -> (array=w42:tag[])
          n34 = call "check_is_empty.vi"("Channels"=w48) -> ("Has Empty?"=w46:bool)
          n35 = call "check_is_empty.vi"("Channels"=w47) -> ("Has Empty?"=w45:bool)
          n36 = call "check_is_empty.vi"("Channels"=w44) -> ("Has Empty?"=w41:bool)
          n37 = call "check_is_empty.vi"("Channels"=w42) -> ("Has Empty?"=w40:bool)
          n38 = Or(x=w46, y=w45) -> (x .or. y?=w43:bool)
          n39 = Or(x=w41, y=w40) -> (x .or. y?=w39:bool)
          n40 = Not Or(1:w39, 2:w43) -> (0:w27:bool)
          n41 = property on="System Running" class="Bool (strict)"("Value"=w27) -> ()  [unwired: 2 in, 2 out]
          n42 = case shown="True" w27 {
            tunnel: [T1."Settings" ("Tab Control") T1."Pressure/Temperature/Offsets" ("Tab Control")] -> w30
            frame False {
              # "Auto Switch to Settings Tab"
            }
            frame True {
              w50 = T21."Disabled and Grayed Out" ("Disabled")
              # "All Settings are valid!"
              n43 = property on="Input" class="Clust (strict)"("DisabledEnum"=w50) -> ()  [unwired: 2 in, 2 out]
              n44 = property on="Output" class="Clust (strict)"("DisabledEnum"=w50) -> ()  [unwired: 2 in, 2 out]
              n45 = property on="Safety" class="Clust (strict)"("DisabledEnum"=w50) -> ()  [unwired: 2 in, 2 out]
            }
          }
          n46 = Not(x=w27) -> (.not. x?=w38:bool)
          n47 = call "Display Message to User5"("Enable"=w38, "Message"="Every line needs a Physical Channel!") -> ("OK"=w36:bool)  [unwired: 8 in, 1 out]
          n48 = Stop(stop? (T)=w36) -> ()
          n49 = property on="Tab Control" class="TabCtl (strict)"("Value"=w30) -> ()  [unwired: 2 in, 2 out]
        }
        frame Disabled {
        }
      }
      n50 = disable-structure shown="Enabled" {
        frame Disabled {
        }
        frame Enabled {
          # "Queue for determining Psat Offsets"
          n51 = Initialize Array(0.0 ("element"), 7 ("dimension size")) -> (w25:dbl[])
          n52 = Obtain Queue(name (unnamed)="autoOffsetPsatQueue", element data type=w25) -> (queue out=→"autoOffsetPsatQueue":refnum<queue>)  [unwired: 3 in, 2 out]
          n53 = Obtain Queue(name (unnamed)="dPDataQueue", element data type=dbl[][] [] ("appended array")) -> (queue out=→"dP Queue":refnum<queue>)  [unwired: 3 in, 2 out]
          n54 = Obtain Queue(name (unnamed)="LoopDataQueue", element data type=T20 {"Vapor Flow rate [g/s]"=0.0, "Liquid Flow rate [g/s]"=0.0, "Pressure/Temperature/Mixture Properties"={"Line Densities\n[g/cm^3]"={"Vapor Line"=0.15445189986836314, "Liquid Line"=0.25755261741892205}, "Mixture Properties"={"Enthalpy"=195841526251804.2, "Quality [-]"=-10.825375459319764}, "[Readings]"={"Streamwise P"=-3074.4228785963764, "Streamwise T"=nan, "Streamwise Sat P"=nan, "Streamwise Sat T"=nan, "Liquid Tank P"=3834985507386.06, "Liquid Tank T"=456.4106234658312, "Liquid Tank Sat P"=1736233577203.0627, "Liquid Tank Sat T"=492.17973224367375, "Separator P"=179910.46497250997, "Separator T"=-13120080.345725078, "Separator Sat P"=0.0, "Separator Sat T"=30.62899308837065, "Liquid Inlet P"=185261.09355383943, "Liquid Inlet T"=508.4593419640114, "Liquid Inlet Sat P"=12378986008470.418, "Liquid Inlet Sat T"=31.430570229281372, "Vapor Tank P"=108956.35947325415, "Vapor Tank T"=-10372083.904135285, "Vapor Tank Sat P"=0.0, "Vapor Tank Sat T"=16.912041354361705, "Vapor Inlet P"=379651.1166364239, "Vapor Inlet T"=381.53210552887515, "Vapor Inlet Sat P"=102884868683.01198, "Vapor Inlet Sat T"=51.054688909951395, "Upper Test Section P"=44976.833741485905, "Upper Test Section T"=-16719245.882515587, "Upper Test Section Sat P"=0.0, "Upper Test Section Sat T"=-7.288297090299707, "Lower Test Section P"=4027555317727.7935, "Lower Test Section T"=527.5685201983387, "Lower Test Section Sat P"=25461496462993.004, "Lower Test Section Sat T"=493.51977461723476}, "Condensor/Evaporator\nTemperature"={"Bottom Evaporator\nTemperature [C]"=0.011951520540655883, "Bottom Condensor\nTemperature [C]"=-36481825.305210106, "Top Evaporator\nTemperature [C]"=-0.005944396537208351, "Top Condensor\nTemperature [C]"=-0.03695927054192248}, "Test Section \nPressure [Pa]"=62496.106498599445, "Heater Temperatures [C]"={"Vapor Tank"=0.025136174921612436, "Liquid Tank"=0.021290742477967885}}, "Seconds Since \nSession Start"=0.0} ("output cluster")) -> (queue out=→"loopDataQueue":refnum<queue>)  [unwired: 3 in, 2 out]
        }
      }
    }
    frame #2 {
      # "Watchdog and settings disabling"
      n55 = disable-structure shown="Enabled" {
        disable-tunnel: [w62 _] -> w59
        disable-tunnel: [w61 _] -> w58
        frame Disabled {
          n56 = for {
            tunnel: "Watchdog Configurations" -> [w77] mode=indexing
            tunnel: [w66] -> w62 mode=indexing
            shift-right: [w65] -> w61
            shift-left: errorcluster {"status"=FALSE, "code"=0, "source"=""} ("error constant") -> [w64]
            n57 = Unbundle(w77) -> ("Task Name"=w74:string, "DAQmx Device Name"=w73:tag, "Digital Outputs"=w75:T23, "Analog Outputs"=w71:T24, "Counter Outputs"=w68:T23)
            n58 = call <vilib>:"DAQmx Create Watchdog Timer Task.vi"("device in"=w73, "new task name"=w74, "timeout"=1.0, "error in"=w64, "digital physical channel expiration states"=w75) -> ("task out"=w72:refnum<k21>, "error out"=w67:errorcluster)  [unwired: 9 in]
            n59 = call-poly <vilib>:"DAQmx Configure Watchdog Expiration States.vi"("task in"=w72, "expiration states"=w71, "error in"=w67) -> ("task out"=w70:refnum<k21>, "error out"=w69:errorcluster)  [unwired: 11 in]
            n60 = call-poly <vilib>:"DAQmx Configure Watchdog Expiration States.vi"("task in"=w70, "expiration states"=w68, "error in"=w69) -> ("task out"=w66:refnum<k21>, "error out"=w65:errorcluster)  [unwired: 11 in]
          }
        }
        frame Enabled {
        }
      }
    }
    frame #3 {
      w92 = 1000.0  # sampling rate
      w88 = 200  # number of samples
      # "Setup all measurement channels for the main loop PT sensors"
      n61 = disable-structure shown="Enabled" {
        disable-tunnel: w85 -> [w180 _]
        disable-tunnel: w84 -> [w179 _]
        frame Disabled {
          n62 = while {
            tunnel: w180 -> [w190] mode=indexing
            tunnel: [w187] -> w178 mode=indexing
            shift-right: [w185] -> w177
            shift-left: w179 -> [w189]
            stop <- w186 stop-if-true
            w188 = 0 items=["reset timer", "clear expiration"] ("action")
            n63 = local read "Stop"() -> (w186:bool)
            n64 = call <vilib>:"DAQmx Control Watchdog Task.vi"("task in"=w190, "action"=w188, "error in"=w189) -> ("task out"=w187:refnum<k21>, "error out"=w185:errorcluster)  [unwired: 11 in]
            n65 = Wait (ms)(milliseconds to wait=u32 100) -> ()  [unwired: 1 out]
          }
          n66 = for {
            tunnel: w178 -> [w183] mode=indexing
            shift-right: [w181] -> _
            shift-left: w177 -> [w182]
            n67 = call <vilib>:"DAQmx Clear Task.vi"("task in"=w183, "error in"=w182) -> ("error out"=w181:errorcluster)  [unwired: 13 in]
          }
        }
        frame Enabled {
        }
      }
      n68 = disable-structure shown="Enabled" {
        frame Enabled {
          n69 = global write "Stop_Global_Variable.vi" "Stop"("Record Loop Data") -> ()
          n70 = call "loop_data_labels.vi"() -> ("Loop Data Labels"=→"Loop Data Labels":string[])
          n71 = call "dP_data_labels.vi"() -> ("dP Data Labels"=→"dP Data Labels":string[])
        }
        frame Disabled {
        }
      }
      n72 = local read "Input"() -> (w87:T13)
      n73 = Unbundle By Name(w87) -> ("Test Section Physical Channels"=w86:T10)
      n74 = call "test_section_daqmx_task.vi"("Test Section Physical Channels"=w86, "sampling rate"=w92, "number of samples"=w88) -> ("error out"=w94:errorcluster, "task out"=w95:refnum<k21>)  [unwired: 7 in]
      n75 = Get Date/Time In Seconds "Start Time\nIn Seconds"() -> (seconds since 1Jan1904=w82:timestamp)
      "start time" <- w82
      n76 = Tick Count (ms)() -> (millisecond timer value=w93:u32)
      n77 = local read "loopDataQueue"() -> (w78:refnum<queue>)
      n78 = while {
        stop <- w191 stop-if-true
        # "Disables Setpoint/Voltage for Manual/PID modes"
        n79 = local read "Stop"() -> (w191:bool)
        n80 = event shown="[1] \"Vapor PID Control.Mode\": Value Change" {
          selector: _ -> [_ _ _]
          dyn-events: _ -> [_ _ _]
          timeout: 50 -> [_ _ _]
          event Timeout {
            n81 = event-data() -> ()  [unwired: 1 in, 3 out]
          }
          event Value Change {
            n82 = event-data() -> ("NewVal"=w193:bool)  [unwired: 1 in]
            n83 = case shown="True" w193 {
              frame False {
                n84 = control-ref of="Valve Voltage [V]"() -> (w197:refnum<vi>)
                n85 = property class="DigNum (strict)"(reference=w197, "DisabledEnum"=T21."Enabled" ("Disabled")) -> ()  [unwired: 1 in, 2 out]
                n86 = control-ref of="Flow Set Point [g/s]"() -> (w194:refnum<vi>)
                n87 = property class="DigNum (strict)"(reference=w194, "DisabledEnum"=T21."Disabled and Grayed Out" ("Disabled")) -> ()  [unwired: 1 in, 2 out]
              }
              frame True {
                n88 = property on="Valve Voltage [V]" class="DigNum (strict)"("DisabledEnum"=T21."Disabled and Grayed Out" ("Disabled")) -> ()  [unwired: 2 in, 2 out]
                n89 = property on="Flow Set Point [g/s]" class="DigNum (strict)"("DisabledEnum"=T21."Enabled" ("Disabled")) -> ()  [unwired: 2 in, 2 out]
              }
            }
          }
          event Value Change {
            n90 = event-data() -> ("NewVal"=w200:bool)  [unwired: 1 in]
            n91 = case shown="True" w200 {
              frame False {
                n92 = control-ref of="Valve Voltage [V]"() -> (w204:refnum<vi>)
                n93 = control-ref of="Flow Set Point [g/s]"() -> (w201:refnum<vi>)
                n94 = property class="DigNum (strict)"(reference=w204, "DisabledEnum"=T21."Enabled" ("Disabled")) -> ()  [unwired: 1 in, 2 out]
                n95 = property class="DigNum (strict)"(reference=w201, "DisabledEnum"=T21."Disabled and Grayed Out" ("Disabled")) -> ()  [unwired: 1 in, 2 out]
              }
              frame True {
                n96 = control-ref of="Valve Voltage [V]"() -> (w208:refnum<vi>)
                n97 = control-ref of="Flow Set Point [g/s]"() -> (w205:refnum<vi>)
                n98 = property class="DigNum (strict)"(reference=w208, "DisabledEnum"=T21."Disabled and Grayed Out" ("Disabled")) -> ()  [unwired: 1 in, 2 out]
                n99 = property class="DigNum (strict)"(reference=w205, "DisabledEnum"=T21."Enabled" ("Disabled")) -> ()  [unwired: 1 in, 2 out]
              }
            }
          }
        }
      }
      n100 = disable-structure shown="Enabled" {
        frame Enabled {
          # "Pulse Generator Safety Triggers"
          n101 = local read "Input"() -> (w163:T13)
          n102 = control-ref of="Float 1"() -> (w176:refnum<vi>)
          n103 = control-ref of="Float 2"() -> (w174:refnum<vi>)
          n104 = control-ref of="Float 3"() -> (w173:refnum<vi>)
          n105 = control-ref of="Float 4"() -> (w175:refnum<vi>)
          n106 = Unbundle By Name(w163) -> ("Float Switch Physical Channels"=w165:T11)
          n107 = Build Array(w176, w174, w173, w175) -> (w172:refnum<vi>[])
          n108 = control-ref of="Heater ON?"() -> (w169:refnum<vi>)
          n109 = control-ref of="Absolute Pulse Generator Pressure Limit"() -> (w167:refnum<vi>)
          n110 = control-ref of="Absolute Pulse Generator Temperature Limit"() -> (w162:refnum<vi>)
          n111 = control-ref of="Stop"() -> (w170:refnum<vi>)
          n112 = control-ref of="Seconds Allowed Pulse Generator Excess Pressure"() -> (w166:refnum<vi>)
          n113 = control-ref of="PG Abs"() -> (w168:refnum<vi>)
          n114 = control-ref of="Liquid Temperature"() -> (w161:refnum<vi>)
          n115 = control-ref of="Pulse Generator"() -> (w171:refnum<vi>)
          n116 = Cluster To Array(cluster=w165) -> (array=w164:tag[])
          n117 = call "float_switch_check_debug.vi"("Temperature Refnum"=w161, "Heater Refnum"=w169, "Abs Pressure Refnum"=w168, "Abs Temperature Limit Refnum"=w162, "Timeout Refnum"=w166, "Abs Pressure Limit Refnum"=w167, "STOP! Refnum"=w170, "Pulse Generator Slide Refnum"=w171, "Float Indicator Refnum"=w172, "lines"=w164) -> ()
        }
        frame Disabled {
        }
      }
      n118 = while {
        tunnel: w95 -> [w382]
        tunnel: w94 -> [w381]
        shift-right: [w352] -> _
        shift-left: w93 -> [w353]
        tunnel: w78 -> [w360]
        tunnel: w82 -> [w373]
        tunnel: w88 -> [w349]
        tunnel: [w348] -> w80
        tunnel: [w344] -> w79
        tunnel: [w347] -> _
        i -> [w375]
        stop <- w379 stop-if-true
        w358 = 1000.0  # Timeout [s]
        # "Messiest Calculation subVI"
        n119 = call "loop_time.vi"("previous timer value"=w353) -> ("millisecond timer value"=w352:u32, "Loop Time [ms]"=w346:u32)
        "Loop Time [ms]" <- w346
        n120 = Get Date/Time In Seconds "Iteration\nStart Time"() -> (seconds since 1Jan1904=w374:timestamp)
        "Time Stamp" <- w374
        n121 = local read "Stop"() -> (w379:bool)
        n122 = call "Convert to Dynamic Data3"("Double"=w346) -> ("Dynamic Data Type"=→"Dynamic Data Type":dynamicdata)  [unwired: 3 in]
        n123 = Subtract(x=w374, y=w373) -> (x-y=→"Seconds Since\nSession Start":dbl)
        n124 = call-poly <vilib>:"DAQmx Read.vi"("task/channels in"=w382, "number of samples per channel"=w349, "timeout"=w358, "error in"=w381) -> ("task out"=w344:refnum<k21>, "data"=w359:waveform(dbl)[], "error out"=w348:errorcluster)  [unwired: 9 in]
        n125 = Wait (ms)(milliseconds to wait=u32 0 ("millisecond multiple")) -> ()  [unwired: 1 out]
        n126 = local read "Liquid PID Control"() -> (w369:T6)
        n127 = local read "Vapor PID Control"() -> (w371:T6)
        n128 = local read "Liquid Flow Data"() -> (w377:T5)
        n129 = local read "Vapor Flow Data"() -> (w378:T4)
        n130 = call "main_loop_calculation.vi"("DAQ Data"=w359, "Offset Parameters"="Offset Parameters") -> ("Vapor Flow Data"=w350:T4, "Liquid Flow Data"=w351:T5, "Pressure/Temperature/Mixture Properties"=w357:T2)
        "Pressure/Temperature/Mixture Properties" <- w357
        "Vapor Flow Data" <- w350
        "Liquid Flow Data" <- w351
        n131 = local read "autoOffsetPsatQueue"() -> (w356:refnum<queue>)
        n132 = Unbundle By Name(w369) -> ("Flow Set Point [g/s]"=w367:dbl)
        n133 = local read "Record Loop Data"() -> (w376:bool)
        n134 = Unbundle By Name(w371) -> ("Flow Set Point [g/s]"=w370:dbl)
        n135 = Unbundle By Name(w377) -> ("Liquid Flow rate [g/s]"=w366:dbl)
        n136 = Unbundle By Name(w378) -> ("Vapor Flow rate [g/s]"=w365:dbl)
        n137 = control-ref of="Auto Offset"() -> (w355:refnum<vi>)
        n138 = control-ref of="Auto Offset Progress"() -> (w343:refnum<vi>)
        n139 = case shown="True" w376 {
          tunnel: w357 -> [_ w488]
          tunnel: [w480 w487] -> w347
          tunnel: w360 -> [w480 w483]
          tunnel: w350 -> [_ w482]
          tunnel: w351 -> [_ w481]
          frame False {
          }
          frame True {
            # "Enqueues Test Section Properties"
            n140 = Unbundle By Name(w481) -> ("Liquid Flow rate [g/s]"=w489:dbl)
            n141 = Unbundle By Name(w482) -> ("Vapor Flow rate [g/s]"=w490:dbl)
            n142 = local read "Seconds Since\nSession Start"() -> (w485:dbl)
            n143 = Bundle("Vapor Flow rate [g/s]"=w490, "Liquid Flow rate [g/s]"=w489, "Pressure/Temperature/Mixture Properties"=w488, "Seconds Since\nSession Start"=w485) -> (w484:T25)  [unwired: 1 in]
            n144 = Enqueue Element(queue=w483, element=w484, timeout in ms (-1)=10) -> (queue out=w487:refnum<queue>)  [unwired: 1 in, 2 out]
          }
        }
        n145 = call "enqueue_pressure_auto_offset.vi"("autoOffsetPsatQueue"=w356, "# to average"=20.0, "Auto Offset"=w355, "Pressure/Temperature/Mixture Properties"=w357, "Auto Offset ProgressBar"=w343) -> ()
        n146 = Build Array(w367, w366) -> (w362:dbl[])
        n147 = Build Array(w370, w365) -> (w364:dbl[])
        n148 = call "Convert to Dynamic Data2"("Array"=w362) -> ("Dynamic Data Type"=→"Liquid Mass Flow Rate":dynamicdata)  [unwired: 3 in]
        n149 = call "Convert to Dynamic Data"("Array"=w364) -> ("Dynamic Data Type"=→"Vapor Mass Flow Rate":dynamicdata)  [unwired: 3 in]
        n150 = disable-structure shown="Enabled" {
          disable-tunnel: w351 -> [w434 _]
          disable-tunnel: w350 -> [w433 _]
          frame Enabled {
            w397 = 0.04 ("y")
            w396 = 0.04 ("y")
            n151 = local read "Liquid PID Control"() -> (w405:T6)
            n152 = local read "Vapor PID Control"() -> (w418:T6)
            n153 = Unbundle By Name(w418) -> ("Mode"=w432:bool, "Valve Voltage [V]"=w411:dbl, "Valve On/Off"=w431:bool, "AutoTune"=w401:bool, "proportional gain (Kc)"=w393:dbl, "integral time (Ti, min)"=w392:dbl, "derivative time (Td, min)"=w391:dbl, "Max % Open"=w395:dbl, "Min % Open"=w394:dbl, "Reinitialize?"=w429:bool)
            n154 = Unbundle By Name(w405) -> ("Mode"=w419:bool, "Valve Voltage [V]"=w420:dbl, "Valve On/Off"=w421:bool, "AutoTune"=w402:bool, "proportional gain (Kc)"=w423:dbl, "integral time (Ti, min)"=w389:dbl, "derivative time (Td, min)"=w390:dbl, "Max % Open"=w399:dbl, "Min % Open"=w398:dbl, "Reinitialize?"=w400:bool)
            n155 = Unbundle By Name(w434) -> ("Liquid Flow rate [g/s]"=w422:dbl)
            n156 = Unbundle By Name(w434) -> ("Liquid Flow rate [g/s]"=w403:dbl)
            n157 = Unbundle By Name(w433) -> ("Vapor Flow rate [g/s]"=w410:dbl)
            n158 = Unbundle By Name(w405) -> ("Valve Voltage [V]"=w404:dbl)
            n159 = Multiply(x=w395, y=w396) -> (x*y=w428:dbl)
            n160 = Multiply(x=w396, y=w394) -> (x*y=w427:dbl)
            n161 = Multiply(x=w399, y=w397) -> (x*y=w425:dbl)
            n162 = Multiply(x=w397, y=w398) -> (x*y=w426:dbl)
            n163 = call "max_flow_correlation.vi"("Current Flow Rate"=w410, "Current Voltage"=w411) -> ("Max Flow Rate"=w408:dbl)
            n164 = Bundle("proportional gain (Kc)"=w393, "integral time (Ti, min)"=w392, "derivative time (Td, min)"=w391) -> (w430:T26)  [unwired: 1 in]
            n165 = Bundle("proportional gain (Kc)"=w423, "integral time (Ti, min)"=w389, "derivative time (Td, min)"=w390) -> (w424:T26)  [unwired: 1 in]
            n166 = call "max_flow_correlation.vi"("Current Flow Rate"=w403, "Current Voltage"=w404) -> ("Max Flow Rate"=w407:dbl)
            n167 = control-ref of="Full Flow Rate"() -> (w409:refnum<vi>)
            n168 = case shown="True" w432 {
              tunnel: [w460 w470] -> w415
              tunnel: w411 -> [w469 w476]
              tunnel: w431 -> [w463 w471]
              tunnel: w410 -> [w468 _]
              tunnel: w430 -> [w467 _]
              tunnel: w429 -> [w466 _]
              tunnel: w428 -> [w465 _]
              tunnel: w427 -> [w464 _]
              tunnel: w418 -> [w462 w473]
              tunnel: [w463 w471] -> w416
              tunnel: w401 -> [w459 _]
              frame True {
                n169 = Bundle(w465, w464) -> (w458:cluster{dbl, dbl})  [unwired: 1 in]
                n170 = Add(x=w458, y=1.0) -> (x+y=w457:cluster{dbl, dbl})
                n171 = call <vilib>:"PID Autotuning.vi"("autotune? (F)"=w459, "reinitialize? (F)"=w466, "output range"=w457, "PID gains"=w467, "process variable"=w468, "setpoint"=w469) -> ("output"=w460:dbl)  [unwired: 2 in, 3 out]
                n172 = Bundle By Name(cluster=w462, "Valve Voltage [V]"=w460) -> (w461:T6)
                n173 = local write "Vapor PID Control"(w461) -> ()
              }
              frame False {
                # "1. Valve voltage has to be between 1-5V.\n2. If Valve is off, set to 1V."
                n174 = In Range and Coerce(upper limit=5.0, x=w476, lower limit=1.0) -> (coerced(x)=w470:dbl)  [unwired: 1 out]
                n175 = Bundle By Name(cluster=w473, "Valve Voltage [V]"=w470) -> (w472:T6)
                n176 = local write "Vapor PID Control"(w472) -> ()
              }
            }
            n177 = case shown="False" w419 {
              tunnel: [w440 w449] -> w414
              tunnel: w420 -> [w448 w452]
              tunnel: w421 -> [w442 w450]
              tunnel: w422 -> [w447 _]
              tunnel: w424 -> [w446 _]
              tunnel: w400 -> [w445 _]
              tunnel: w425 -> [w444 _]
              tunnel: w426 -> [w443 _]
              tunnel: w405 -> [w441 w451]
              tunnel: [w442 w450] -> w412
              tunnel: w402 -> [w438 _]
              frame True {
                n178 = Bundle(w444, w443) -> (w437:cluster{dbl, dbl})  [unwired: 1 in]
                n179 = Add(x=w437, y=1.0) -> (x+y=w435:cluster{dbl, dbl})
                n180 = call <vilib>:"PID Autotuning.vi"("autotune? (F)"=w438, "reinitialize? (F)"=w445, "output range"=w435, "PID gains"=w446, "process variable"=w447, "setpoint"=w448) -> ("output"=w440:dbl)  [unwired: 2 in, 3 out]
                n181 = Bundle By Name(cluster=w441, "Valve Voltage [V]"=w440) -> (w439:T6)
                n182 = local write "Liquid PID Control"(w439) -> ()
              }
              frame False {
                # "1. Valve voltage has to be between 1-5V.\n2. If Valve is off, set to 1V."
                n183 = In Range and Coerce(upper limit=5.0, x=w452, lower limit=1.0) -> (coerced(x)=w449:dbl)  [unwired: 1 out]
                n184 = Bundle By Name(cluster=w451, "Valve Voltage [V]"=w449) -> (w455:T6)
                n185 = local write "Liquid PID Control"(w455) -> ()
              }
            }
            n186 = control-ref of="Full Flow Rate"() -> (w406:refnum<vi>)
            n187 = property class="DigNum (strict)"(reference=w409, "Value"=w408) -> ()  [unwired: 1 in, 2 out]
            n188 = property class="DigNum (strict)"(reference=w406, "Value"=w407) -> ()  [unwired: 1 in, 2 out]
            n189 = local read "Output"() -> (w383:T16)
            n190 = Unbundle By Name(w383) -> ("Vapor/Liquid Valve Physical Channels.Vapor Valve"=w385:tag, "Vapor/Liquid Valve Physical Channels.Liquid Valve"=w384:tag)
            n191 = Select(t=w415, s=w416, f=1.0) -> (s? t:f=w388:dbl)
            n192 = Select(t=w414, s=w412, f=1.0) -> (s? t:f=w387:dbl)
            n193 = Build Array(w388, w387) -> (w386:dbl[])
            n194 = call "valve_control_output.vi"("Voltages"=w386, "Liquid channel"=w384, "Vapor channel"=w385) -> ()  [unwired: 1 in]
          }
          frame Disabled {
          }
        }
        n195 = disable-structure shown="Disabled" {
          frame Disabled {
            n196 = call "Vapor Valve Voltage [V]"() -> ("DC"=w479:dynamicdata)  [unwired: 14 in, 1 out]
            n197 = call "Liquid Valve Voltage [V]"() -> ("DC"=w478:dynamicdata)  [unwired: 14 in, 1 out]
            n198 = Merge Signals(w479, w478) -> (w477:dynamicdata)
            n199 = call "DAQ Assistant"("data"=w477) -> ()  [unwired: 17 in, 2 out]
          }
          frame Enabled {
          }
        }
        "# of Averages Processed" <- w375
      }
      n200 = disable-structure shown="Enabled" {
        frame Enabled {
          w140 = T27 {"Pulse Generator to Test Section dP"=refnum, "Pitot dP"=refnum, "Abs Tank Pressure"=refnum, "Camera Voltage"=refnum}  # Pulse Generator Chart Refnums
          w153 = T28 {"Vapor Temperature"=refnum, "Vapor Sat Pressure"=refnum, "Liquid Temperature"=refnum, "Liquid Sat Pressure"=refnum, "PG to TS dP"=refnum, "Pitot Current"=refnum, "Pitot dP"=refnum, "Mass Flow Rate"=refnum, "PG Abs Pressure"=refnum, "W1-4 dP"=refnum, "W1-7 dP"=refnum}  # Pulse Generator Measurement Refnums
          w160 = T29 {"PG Abs Offset"=refnum, "Pitot Offset"=refnum, "PG-TS Offset"=refnum, "Recording Duration"=refnum, "Sampling Rate"=refnum}  # Pulse Generator Offsets and Data Saving Controls Refnums
          # "Everything in the Pulse Generator Data Tab"
          n201 = control-ref of="Pitot dP"() -> (w141:refnum<vi>)
          n202 = control-ref of="Mass Flow Rate"() -> (w151:refnum<vi>)
          n203 = control-ref of="PG Abs"() -> (w150:refnum<vi>)
          n204 = control-ref of="W1-4 dP[Pa]"() -> (w149:refnum<vi>)
          n205 = control-ref of="W1-7 dP[Pa]"() -> (w148:refnum<vi>)
          n206 = control-ref of="Vapor Temperature"() -> (w139:refnum<vi>)
          n207 = control-ref of="Vapor Sat Pressure"() -> (w138:refnum<vi>)
          n208 = control-ref of="Liquid Temperature"() -> (w137:refnum<vi>)
          n209 = control-ref of="Liquid Sat Pressure"() -> (w136:refnum<vi>)
          n210 = control-ref of="PG to TS dP"() -> (w135:refnum<vi>)
          n211 = control-ref of="Pitot Amps"() -> (w134:refnum<vi>)
          n212 = control-ref of="Pulse Generator to Test Section dP"() -> (w147:refnum<vi>)
          n213 = control-ref of="Pitot dP"() -> (w146:refnum<vi>)
          n214 = control-ref of="Absolute Tank Pressure"() -> (w133:refnum<vi>)
          n215 = control-ref of="Camera Voltage"() -> (w132:refnum<vi>)
          n216 = Bundle By Name(cluster=w153, "Vapor Temperature"=w139, "Vapor Sat Pressure"=w138, "Liquid Temperature"=w137, "Liquid Sat Pressure"=w136, "PG to TS dP"=w135, "Pitot Current"=w134, "Pitot dP"=w141, "Mass Flow Rate"=w151, "PG Abs Pressure"=w150, "W1-4 dP"=w149, "W1-7 dP"=w148) -> (w152:T28)
          n217 = control-ref of="PG Abs Offset"() -> (w159:refnum<vi>)
          n218 = control-ref of="Pitot Offset"() -> (w158:refnum<vi>)
          n219 = control-ref of="PG-TS Offset"() -> (w157:refnum<vi>)
          n220 = control-ref of="Recording Duration"() -> (w156:refnum<vi>)
          n221 = control-ref of="Sampling\nFrequency"() -> (w155:refnum<vi>)
          n222 = Bundle By Name(cluster=w140, "Pulse Generator to Test Section dP"=w147, "Pitot dP"=w146, "Abs Tank Pressure"=w133, "Camera Voltage"=w132) -> (w142:T27)
          n223 = Bundle By Name(cluster=w160, "PG Abs Offset"=w159, "Pitot Offset"=w158, "PG-TS Offset"=w157, "Recording Duration"=w156, "Sampling Rate"=w155) -> (w154:T29)
          n224 = local read "start time"() -> (w131:timestamp)
          n225 = control-ref of="Stop"() -> (w143:refnum<vi>)
          n226 = control-ref of="Record dP Data"() -> (w145:refnum<vi>)
          n227 = control-ref of="dP Recording Progress"() -> (w144:refnum<vi>)
          n228 = local read "dP Queue"() -> (w130:refnum<queue>)
          n229 = call "pulse_generator_data.vi"("Record dP Data"=w145, "queue in"=w130, "Stop! Refnum"=w143, "Recording Progressbar"=w144, "Seesion Start Time"=w131, "Pulse Generator Chart Refnums"=w142, "Pulse Generator Offsets and Data Saving Controls Refnums"=w154, "Pulse Generator Measurement Refnums"=w152) -> ()  [unwired: 4 in]
        }
        frame Disabled {
        }
      }
      n230 = while {
        stop <- w210 stop-if-true
        # "Dequeue loop for auto offset function"
        n231 = event shown="[1] \"Auto Offset\": Value Change" {
          selector: _ -> [_ _]
          dyn-events: _ -> [_ _]
          timeout: 10 -> [_ _]
          event Timeout {
            n232 = event-data() -> ()  [unwired: 1 in, 3 out]
          }
          event "Auto Offset": Value Change {
            n233 = event-data() -> ("NewVal"=w211:bool)  [unwired: 1 in]
            n234 = case shown="False" w211 {
              frame False {
                n235 = Initialize Array(0.0 ("element"), 7 ("dimension size")) -> (w233:dbl[])
                n236 = local read "autoOffsetPsatQueue"() -> (w238:refnum<queue>)
                n237 = while {
                  tunnel: w238 -> [w246]
                  shift-right: [w241] -> w237
                  shift-left: w233 -> [w242]
                  tunnel: [w240] -> w235
                  i -> [w240]
                  stop <- w244 stop-if-true
                  n238 = Dequeue Element(queue=w246, timeout in ms (-1)=100) -> (element=w243:dbl[], timed out?=w245:bool)  [unwired: 1 in, 2 out]
                  n239 = case shown="False" w245 {
                    selector: w245 -> [_ w254]
                    tunnel: [w247 w254] -> w244
                    tunnel: w243 -> [w251 _]
                    tunnel: [w250 w253] -> w241
                    tunnel: w242 -> [w252 w253]
                    frame False {
                      n240 = local read "Stop"() -> (w248:bool)
                      n241 = Add(x=w252, y=w251) -> (x+y=w250:dbl[])
                      n242 = Or(x=w248, y=FALSE) -> (x .or. y?=w247:bool)
                    }
                    frame True {
                    }
                  }
                }
                n243 = local read "Offset Parameters"() -> (w220:T3)
                n244 = Add(x=w235, y=1) -> (x+y=w236:i32)
                n245 = Divide(x=w237, y=w236) -> (x/y=w222:dbl[])
                n246 = Unbundle By Name(w220) -> ("Liquid Tank\nPressure"=w219:dbl, "Separator Pressure"=w218:dbl, "Liquid Inlet\nPressure"=w217:dbl, "Vapor Tank\nPressure"=w216:dbl, "Dev Section\nPressure"=w215:dbl, "Upper Test Section\nPressure"=w214:dbl, "Lower Test Section\nPressure"=w213:dbl)
                n247 = Build Array(w219, w218, w217, w216, w215, w214, w213) -> (w212:dbl[])
                n248 = Subtract(x=w222, y=w212) -> (x-y=w221:dbl[])
                n249 = Index Array(array=w221) -> (element #1=w229:dbl, element #2=w228:dbl, element #3=w227:dbl, element #4=w226:dbl, element #5=w225:dbl, element #6=w224:dbl, element #7=w223:dbl)  [unwired: 7 in]
                n250 = Bundle By Name(cluster=w220, "Liquid Tank\nPressure"=w229, "Separator Pressure"=w228, "Liquid Inlet\nPressure"=w227, "Vapor Tank\nPressure"=w226, "Dev Section\nPressure"=w225, "Upper Test Section\nPressure"=w224, "Lower Test Section\nPressure"=w223) -> (w230:T3)
                n251 = local write "Offset Parameters"(w230) -> ()
              }
              frame True {
              }
            }
          }
        }
        n252 = local read "Stop"() -> (w210:bool)
      }
      n253 = disable-structure shown="Enabled" {
        frame Disabled {
        }
        frame Enabled {
          w108 = T30 {"Start Pulse"=refnum, "Stop Pulse"=refnum, "Heaters"=refnum, "Counter"=refnum, "Frequency (Hz)"=refnum, "Duty Cycle"=refnum, "Idle State"=refnum, "Pulse Generator Active"=refnum, "Stepper Motor Direction"=refnum, "Steps"=refnum, "Direction Line"=refnum, "1000-1 Line"=refnum, "1000-2 Line"=refnum, "1000-3 Line"=refnum, "500-1 Line"=refnum, "250-1 Line"=refnum, "125-1 Line Var"=refnum, "1000-1"=refnum, "1000-2"=refnum, "1000-3"=refnum, "500-1"=refnum, "250-1"=refnum, "125-1"=refnum, "125W Frequency (Hz)"=refnum, "125W Duty Cycle"=refnum, "Heater ON?"=refnum, "125-1 Line Fix"=refnum}  # Pulse Generator Control Refnums
          # "Controls Heaters and Stepper Motor, listens to stopping signals."
          n254 = control-ref of="125W 1 Fix"() -> (w107:refnum<vi>)
          n255 = control-ref of="Counter Line"() -> (w115:refnum<vi>)
          n256 = control-ref of="Direction Line"() -> (w118:refnum<vi>)
          n257 = control-ref of="1000W 1"() -> (w122:refnum<vi>)
          n258 = control-ref of="1000W 2"() -> (w128:refnum<vi>)
          n259 = control-ref of="1000W 3"() -> (w123:refnum<vi>)
          n260 = control-ref of="500W 1"() -> (w124:refnum<vi>)
          n261 = control-ref of="250W 1"() -> (w125:refnum<vi>)
          n262 = control-ref of="125W 1 Var"() -> (w112:refnum<vi>)
          n263 = control-ref of="Start Pulse"() -> (w117:refnum<vi>)
          n264 = control-ref of="Stop Pulse"() -> (w116:refnum<vi>)
          n265 = control-ref of="Heater ON?"() -> (w110:refnum<vi>)
          n266 = control-ref of="Pulse Gen Active?"() -> (w113:refnum<vi>)
          n267 = control-ref of="Heaters"() -> (w111:refnum<vi>)
          n268 = control-ref of="1000-2"() -> (w121:refnum<vi>)
          n269 = control-ref of="1000-1"() -> (w127:refnum<vi>)
          n270 = control-ref of="1000-2"() -> (w126:refnum<vi>)
          n271 = control-ref of="1000-3"() -> (w129:refnum<vi>)
          n272 = control-ref of="500-1"() -> (w106:refnum<vi>)
          n273 = control-ref of="250-1"() -> (w105:refnum<vi>)
          n274 = control-ref of="125-1"() -> (w104:refnum<vi>)
          n275 = control-ref of="Frequency (Hz)"() -> (w114:refnum<vi>)
          n276 = control-ref of="Duty Cycle"() -> (w101:refnum<vi>)
          n277 = control-ref of="Steps"() -> (w100:refnum<vi>)
          n278 = control-ref of="125W Frequency (Hz)"() -> (w103:refnum<vi>)
          n279 = control-ref of="125W Duty Cycle"() -> (w102:refnum<vi>)
          n280 = control-ref of="Idle State"() -> (w99:refnum<vi>)
          n281 = Bundle By Name(cluster=w108, "Start Pulse"=w117, "Stop Pulse"=w116, "Heaters"=w110, "Counter"=w115, "Frequency (Hz)"=w114, "Duty Cycle"=w101, "Steps"=w100, "Idle State"=w99, "Pulse Generator Active"=w113, "Stepper Motor Direction"=w111, "Direction Line"=w118, "Heater ON?"=w121, "1000-1 Line"=w122, "1000-2 Line"=w128, "1000-3 Line"=w123, "500-1 Line"=w124, "250-1 Line"=w125, "125-1 Line Var"=w112, "125-1 Line Fix"=w107, "1000-1"=w127, "1000-2"=w126, "1000-3"=w129, "500-1"=w106, "250-1"=w105, "125-1"=w104, "125W Frequency (Hz)"=w103, "125W Duty Cycle"=w102) -> (w119:T30)
          n282 = control-ref of="125W Variable/Fixed"() -> (w109:refnum<vi>)
          n283 = control-ref of="Stop"() -> (w120:refnum<vi>)
          n284 = call "pulse_generator_multiheater_refnum.vi"("125W Fixed/Variable"=w109, "Stop! Refnum"=w120, "Pulse Generator Control Multiheater Refnums"=w119) -> ()  [unwired: 1 in]
        }
      }
      n285 = local read "dP Queue"() -> (w83:refnum<queue>)
      n286 = while {
        tunnel: w83 -> [w256]
        stop <- w255 stop-if-true
        # "Makes sure the path and daq settings cannot be changed while data is being recorded."
        n287 = event shown="[1] \"Record dP Data\": Value Change" {
          selector: _ -> [_ _]
          dyn-events: _ -> [_ _]
          timeout: 10 -> [_ _]
          tunnel: w256 -> [_ w259]
          event Timeout {
            n288 = event-data() -> ()  [unwired: 1 in, 3 out]
          }
          event "Record dP Data": Value Change {
            n289 = event-data() -> ("NewVal"=w258:bool)  [unwired: 1 in, 5 out]
            n290 = case shown="False" w258 {
              tunnel: w259 -> [w260 _]
              frame False {
                n291 = flat-sequence {
                  tunnel: w260 -> [w261]
                  frame #0 {
                    n292 = while {
                      tunnel: w261 -> [w262]
                      stop <- w263 stop-if-true
                      n293 = Get Queue Status(queue=w262) -> (# elements in queue=w267:i32)  [unwired: 2 in, 7 out]
                      n294 = local read "Stop"() -> (w264:bool)
                      n295 = Equal?(x=0, y=w267) -> (x = y?=w265:bool)
                      n296 = Or(x=w265, y=w264) -> (x .or. y?=w263:bool)
                    }
                  }
                  frame #1 {
                    n297 = Wait (ms)(milliseconds to wait=u32 100) -> ()  [unwired: 1 out]
                  }
                  frame #2 {
                    w269 = T21."Enabled" ("Disabled")
                    n298 = local read "dP Data Index"() -> (w279:dbl)
                    n299 = control-ref of="dP Data Folder"() -> (w277:refnum<vi>)
                    n300 = control-ref of="dP Data Prefix"() -> (w274:refnum<vi>)
                    n301 = property class="Path"(reference=w277, "DisabledEnum"=T21."Enabled" ("Disabled")) -> ()  [unwired: 1 in, 2 out]
                    n302 = property class="Str"(reference=w274, "DisabledEnum"=T21."Enabled" ("Disabled")) -> ()  [unwired: 1 in, 2 out]
                    n303 = Add(x=w279, y=1.0) -> (x+y=w278:dbl)
                    n304 = local write "dP Data Index"(w278) -> ()
                    n305 = control-ref of="Recording Duration"() -> (w272:refnum<vi>)
                    n306 = control-ref of="Sampling Frequency"() -> (w271:refnum<vi>)
                    n307 = control-ref of="Record dP Data"() -> (w273:refnum<vi>)
                    n308 = property class="Bool (strict)"(reference=w273, "DisabledEnum"=w269) -> ()  [unwired: 1 in, 2 out]
                    n309 = property class="DigNum (strict)"(reference=w272, "DisabledEnum"=w269) -> ()  [unwired: 1 in, 2 out]
                    n310 = property class="DigNum (strict)"(reference=w271, "DisabledEnum"=w269) -> ()  [unwired: 1 in, 2 out]
                  }
                }
              }
              frame True {
                n311 = control-ref of="dP Data Folder"() -> (w295:refnum<vi>)
                n312 = control-ref of="Recording Duration"() -> (w289:refnum<vi>)
                n313 = control-ref of="Record dP Data"() -> (w290:refnum<vi>)
                n314 = property class="Path"(reference=w295, "DisabledEnum"=T21."Disabled and Grayed Out" ("Disabled")) -> ()  [unwired: 1 in, 2 out]
                n315 = property class="Bool (strict)"(reference=w290, "DisabledEnum"=T21."Disabled and Grayed Out" ("Disabled")) -> ()  [unwired: 1 in, 2 out]
                n316 = property class="DigNum (strict)"(reference=w289, "DisabledEnum"=T21."Disabled and Grayed Out" ("Disabled")) -> ()  [unwired: 1 in, 2 out]
                n317 = control-ref of="Sampling\nFrequency"() -> (w286:refnum<vi>)
                n318 = control-ref of="dP Data Prefix"() -> (w292:refnum<vi>)
                n319 = property class="Str"(reference=w292, "DisabledEnum"=T21."Disabled and Grayed Out" ("Disabled")) -> ()  [unwired: 1 in, 2 out]
                n320 = property class="DigNum (strict)"(reference=w286, "DisabledEnum"=T21."Disabled and Grayed Out" ("Disabled")) -> ()  [unwired: 1 in, 2 out]
                n321 = control-ref of="Recording Duration"() -> (w284:refnum<vi>)
                n322 = control-ref of="dP Recording Progress"() -> (w285:refnum<vi>)
                n323 = control-ref of="Sampling\nFrequency"() -> (w283:refnum<vi>)
                n324 = property class="DigNum (strict)"(reference=w284) -> ("Value"=w282:dbl)  [unwired: 1 in, 2 out]
                n325 = property class="DigNum (strict)"(reference=w283) -> ("Value"=w281:dbl)  [unwired: 1 in, 2 out]
                n326 = Multiply(x=w282, y=w281) -> (x*y=w280:dbl)
                n327 = property class="Slide (strict)"(reference=w285, "Scale.Maximum"=w280) -> ()  [unwired: 1 in, 2 out]
              }
            }
          }
        }
        n328 = local read "Stop"() -> (w255:bool)
      }
      n329 = while {
        tunnel: w83 -> [w302]
        tunnel: [w298] -> _
        tunnel: [w297] -> _
        stop <- w299 stop-if-true
        # "Dequeue loop of dP-data logging"
        n330 = Dequeue Element(queue=w302, timeout in ms (-1)=50) -> (queue out=w298:refnum<queue>, element=w300:dbl[][], timed out?=w296:bool, error out=w297:errorcluster)  [unwired: 1 in]
        n331 = case shown="False" w296 {
          tunnel: w300 -> [w303 _]
          frame False {
            n332 = local read "dP Data Labels"() -> (w304:string[])
            n333 = local read "dP Data Prefix"() -> (w306:string)
            n334 = local read "dP Data Folder"() -> (w307:path)
            n335 = local read "dP Data Index"() -> (w305:dbl)
            n336 = call "write_dp_data.vi"("dequeued data"=w303, "dP Data Labels"=w304, "dP Data Index"=w305, "dP Data Prefix"=w306, "dP Data Folder"=w307) -> ()
          }
          frame True {
          }
        }
        n337 = local read "Stop"() -> (w299:bool)
      }
      n338 = local read "loopDataQueue"() -> (w81:refnum<queue>)
      n339 = while {
        tunnel: w81 -> [w309]
        stop <- w308 stop-if-true
        # "Makes sure the path cannot be changed while data is being recorded."
        n340 = event shown="[1] \"Record Loop Data\": Value Change" {
          selector: _ -> [_ _]
          dyn-events: _ -> [_ _]
          timeout: 10 -> [_ _]
          tunnel: w309 -> [_ w311]
          event Timeout {
            n341 = event-data() -> ()  [unwired: 1 in, 3 out]
          }
          event "Record Loop Data": Value Change {
            n342 = event-data() -> ("NewVal"=w312:bool)  [unwired: 1 in, 4 out]
            n343 = case shown="False" w312 {
              tunnel: w311 -> [w313 _]
              frame False {
                n344 = flat-sequence {
                  tunnel: w313 -> [w314]
                  frame #0 {
                    n345 = while {
                      tunnel: w314 -> [w320]
                      stop <- w315 stop-if-true
                      n346 = Get Queue Status(queue=w320) -> (# elements in queue=w319:i32)  [unwired: 2 in, 7 out]
                      n347 = Equal?(x=0, y=w319) -> (x = y?=w317:bool)
                      n348 = local read "Stop"() -> (w316:bool)
                      n349 = Or(x=w317, y=w316) -> (x .or. y?=w315:bool)
                    }
                  }
                  frame #1 {
                    n350 = Wait (ms)(milliseconds to wait=u32 100) -> ()  [unwired: 1 out]
                  }
                  frame #2 {
                    n351 = control-ref of="Loop Data Prefix"() -> (w322:refnum<vi>)
                    n352 = local read "Loop Data Index"() -> (w328:dbl)
                    n353 = property class="Str"(reference=w322, "DisabledEnum"=T21."Enabled" ("Disabled")) -> ()  [unwired: 1 in, 2 out]
                    n354 = control-ref of="Loop Data Folder"() -> (w325:refnum<vi>)
                    n355 = Add(x=w328, y=1.0) -> (x+y=w326:dbl)
                    n356 = local write "Loop Data Index"(w326) -> ()
                    n357 = property class="Path"(reference=w325, "DisabledEnum"=T21."Enabled" ("Disabled")) -> ()  [unwired: 1 in, 2 out]
                  }
                }
              }
              frame True {
                n358 = control-ref of="Loop Data Folder"() -> (w332:refnum<vi>)
                n359 = control-ref of="Loop Data Prefix"() -> (w329:refnum<vi>)
                n360 = property class="Str"(reference=w329, "DisabledEnum"=T21."Disabled and Grayed Out" ("Disabled")) -> ()  [unwired: 1 in, 2 out]
                n361 = property class="Path"(reference=w332, "DisabledEnum"=T21."Disabled and Grayed Out" ("Disabled")) -> ()  [unwired: 1 in, 2 out]
              }
            }
          }
        }
        n362 = local read "Stop"() -> (w308:bool)
      }
      n363 = while {
        tunnel: w81 -> [w337]
        stop <- w334 stop-if-true
        # "Dequeue test section-data"
        n364 = local read "Stop"() -> (w334:bool)
        n365 = Dequeue Element(queue=w337, timeout in ms (-1)=50) -> (element=w335:T20, timed out?=w333:bool)  [unwired: 1 in, 2 out]
        n366 = case shown="False" w333 {
          tunnel: w335 -> [w338 _]
          frame False {
            n367 = local read "Loop Data Folder"() -> (w342:path)
            n368 = local read "Loop Data Labels"() -> (w339:string[])
            n369 = local read "Loop Data Prefix"() -> (w341:string)
            n370 = local read "Loop Data Index"() -> (w340:dbl)
            n371 = call "write_test_section_data.vi"("dequeued data"=w338, "Loop Data Labels"=w339, "Loop Data Index"=w340, "Loop Data Prefix"=w341, "Loop Data Folder"=w342) -> ()
          }
          frame True {
          }
        }
      }
      n372 = call <vilib>:"DAQmx Stop Task.vi"("task/channels in"=w79, "error in"=w80) -> ("task out"=w89:refnum<k21>, "error out"=w90:errorcluster)  [unwired: 12 in]
      n373 = call <vilib>:"DAQmx Clear Task.vi"("task in"=w89, "error in"=w90) -> ("error out"=w91:errorcluster)  [unwired: 13 in]
    }
    frame #4 {
      w491 = T21."Enabled" ("Disabled")
      n374 = Merge Errors(w492) -> (→"error out":errorcluster)
      n375 = control-ref of="Stop"() -> (w497:refnum<vi>)
      n376 = control-ref of="System Running"() -> (w494:refnum<vi>)
      n377 = property class="Bool (strict)"(reference=w497, "Value"=FALSE) -> ()  [unwired: 1 in, 2 out]
      n378 = property class="Bool (strict)"(reference=w494, "Value"=FALSE) -> ()  [unwired: 1 in, 2 out]
      n379 = property on="Input" class="Clust (strict)"("DisabledEnum"=w491) -> ()  [unwired: 2 in, 2 out]
      n380 = property on="Safety" class="Clust (strict)"("DisabledEnum"=w491) -> ()  [unwired: 2 in, 2 out]
      n381 = property on="Output" class="Clust (strict)"("DisabledEnum"=w491) -> ()  [unwired: 2 in, 2 out]
    }
  }
